vi "Lockin_sweep.vi"(0 "Transport":refnum<class "Transport.lvclass">, 3 "error in (no error)":errorcluster) -> (7 "Transport out":refnum<class "Transport.lvclass">, 10 "error out":errorcluster)   [LabVIEW 2019, in "Transport.lvclass"]
doc: "This VI uses the Lockin Sweep Method. That is, you tell the lockin to sweep from Start to End in a certain amount of time. The lockin will run independently while it executes the sweep. While the lockin is sweeping, this VI will poll the lockin once per second to get a snapshot of current results and the sweep status (sweeping or not sweeping). When the lockin is finished sweeping this VI will ask for the final sweep results and save them. The spacing between points is determined by the \"Fs Output\" control in the Lockin."
uses:
  Transport.lvclass
  Control Experiment/Control Experiment.lvclass
  <userlib>/LevyLab/Lockin-Multichannel/Instrument.DAQ/Typedefs/Sweep.Configuration--Cluster.ctl
  <userlib>/LevyLab/Lockin-Multichannel/Instrument.DAQ/Instrument.DAQ.lvclass
  <userlib>/LevyLab/Lockin-Multichannel/Instrument.DAQ/Typedefs/Sweep.Channel--Cluster.ctl
  <userlib>/LevyLab/Lockin-Multichannel/Instrument.Lockin/Instrument.Lockin.lvclass
  <userlib>/LevyLab/Lockin-Multichannel/Instrument.Lockin/Typedefs/Results Type--Enum.ctl
  <userlib>/LevyLab/Lockin-Multichannel/Instrument.DAQ/Typedefs/Sweep.Pattern--Enum.ctl
  <userlib>/LevyLab/Lockin-Multichannel/Instrument.DAQ/Typedefs/Sweep.Channel--Cluster--Array.ctl
  <vilib>/PRIrvin/XY Utilities/xy_utilities.lvlib
  217905a9-ad64-4e54-8703-31da4ffbd4c0.vi
  9896b5e5-a649-4b1b-acc0-fd49b17a1bc1.vi
  Typedefs/Lockin_Sweep JSON--Cluster.ctl
  <userlib>/LevyLab/Instrument Framework/Instrument Types/Cryostat/Typedefs/Magnet Axis--Enum.ctl
  <userlib>/LevyLab/Instrument Framework/Instrument Types/Cryostat/Instrument.Cryostat.lvclass
  <userlib>/LevyLab/Instrument Framework/Instrument Types/CBridge/Instrument.CBridge.lvclass
  <userlib>/LevyLab/Instrument Framework/Instrument Types/Strain/Instrument.Strain.lvclass
  C:/Program Files/National Instruments/LabVIEW 2019/user.lib/LevyLab/Instrument Framework/Instrument/Instrument.lvclass
  C:/Program Files/National Instruments/LabVIEW 2019/vi.lib/JKI/JKI SMO/SMO/SMO.lvclass
  <vilib>/PRIrvin/XY Utilities/subVIs/Divide float (multiple).vi
  <vilib>/PRIrvin/XY Utilities/subVIs/Multiply float (multiple).vi
  <vilib>/Utility/Data Type/NI_Data Type.lvlib
  <userlib>/LevyLab/Instrument Framework/Instrument/Instrument.lvclass
  <userlib>/LevyLab/Instrument Framework/Instrument Types/Lockin/Instrument.LockinAPI.lvclass
  <userlib>/LevyLab/Instrument Framework/Instrument Types/Amplifier/Instrument.Amplifier.lvclass
  <userlib>/LevyLab/Instrument Framework/Instrument Types/Delay Line/Instrument.DelayLine.lvclass
  <userlib>/LevyLab/Instrument Framework/Instrument Types/VNA/Instrument.VNA.lvclass
  <userlib>/LevyLab/Instrument Framework/Instrument Types/VSource/Instrument.VSource.lvclass
  Control Experiment/Typedefs/Instrument Types--enum.ctl
  Attributes/Instrument Attributes.lvlib
  ac72d6f7-f5c3-431a-8621-5120436d0f52.vi
  <userlib>/LevyLab/Debug/Debug.lvlib
  d7da78e6-7697-4005-8475-e4e7ed229128.vi
  C:/Program Files/National Instruments/LabVIEW 2019/user.lib/LevyLab/Instrument Framework/Instrument Types/Lockin/Instrument.LockinAPI.lvclass
panel:
  in  "stop":bool
  in  "Tab Control":T1(tab)
  in  "refresh (ms)":u32=1000
  out "state history":string
  out "Sweep Tables":cluster{"Ch":i32, "Table":dbl[]}[](array[cluster]) {"Table" format="%#_3p"; "Ch" min=1 max=16}
  in  "Emergency Stop Visible?":bool
  out "elapsed time (s)":i32=231
  out "Experiment Comments":string
  out "Experiment Folder":string
  out "time b/w points (ms)":u32=1037
  out "Sweep Channels":T2 {"Table" format="%#_1f"; "Channel" min=1 max=128; "Start" format="%#_6p"; "End" format="%#_6p"}
  out "Sweep Time (s)":dbl
  out "Initial Wait (s)":dbl
  out "Return to Start":bool
  out "Instrument Status":string
  in  "Emergency Stop 1":bool caption="Emergency Stop"
  out "Lockin (X)":cluster{"Wavenumber":dbl[], "Data":dbl[]}[](graph)
  out "Lockin (Y)":cluster{"Wavenumber":dbl[], "Data":dbl[]}[](graph)
  in  "Units":enum16{"ohms & siemens", "h/e2 & e2/h"}(ring)
  out "Resistance":cluster{"X-array":dbl[], "Y-array":dbl[]}[](graph)
  out "Conductance":cluster{"X-array":dbl[], "Y-array":dbl[]}[](graph)
  in  "Emergency Stop 2":bool caption="Emergency Stop"
  out "AI":cluster{"Wavenumber":dbl[], "Data":dbl[]}[](graph)
  out "AO":cluster{"Wavenumber":dbl[], "Data":dbl[]}[](graph)
  in  "Emergency Stop 3":bool caption="Emergency Stop"
  out "2 Terminal":cluster{"Wavenumber":dbl[], "Data":dbl[]}[](graph)
  out "4 Terminal":cluster{"Wavenumber":dbl[], "Data":dbl[]}[](graph)
  in  "Emergency Stop 4":bool caption="Emergency Stop"
  # "VI Configuration"
  # "Status"
  # "Experiment Configuration*"
  # "VI Description"
  # "Run a sweep on the lockin itself. The lockin is told to sweep from Start to End over a set time, and it runs the sweep on its own. While it sweeps, this VI polls the lockin once per fresh time for a snapshot of the current results and the sweep status. When the sweep finishes, it reads the final sweep results and saves them. The point spacing is set by the lockin's \"Fs Output\" control."
  # "*Change these values in Transport Server"
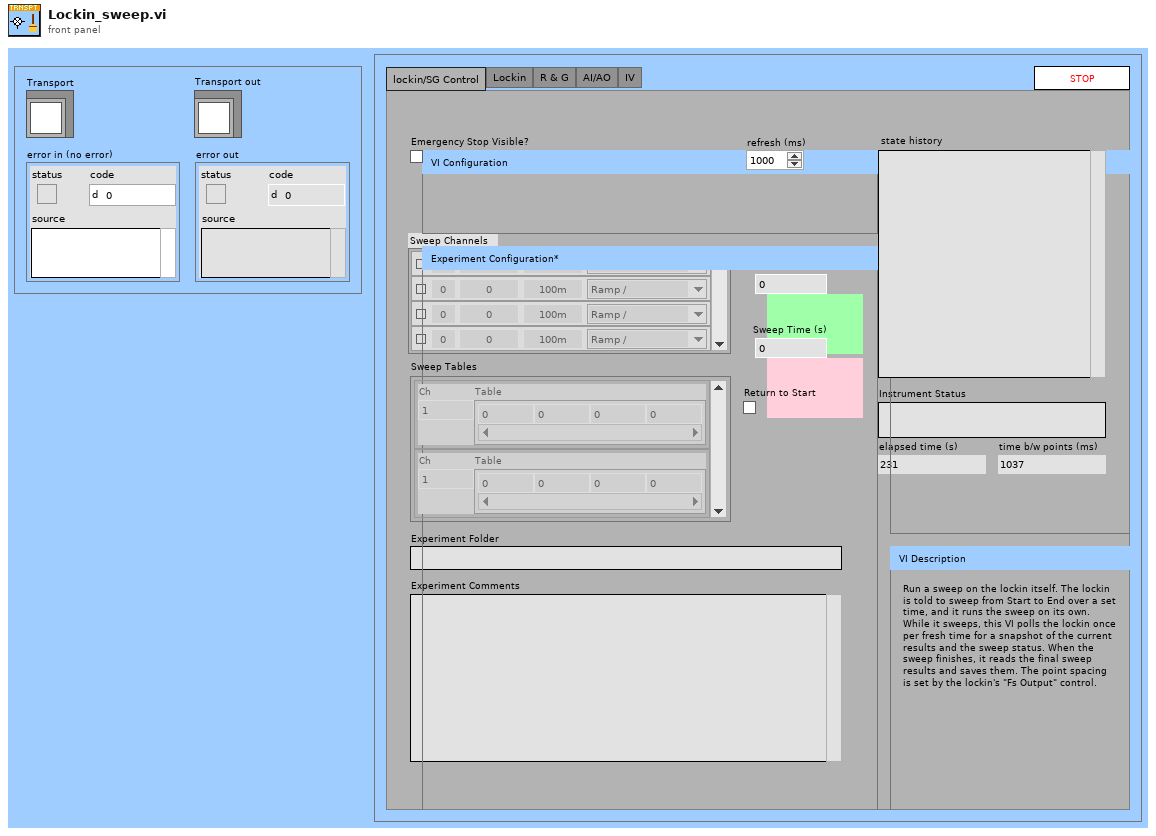
[diagram p1: front panel]
types:
  T1 = enum32{"lockin/SG Control", "Lockin", "R & G", "AI/AO", "IV"}
  T2 = typedef "Instrument.Lockin.lvlib/Instrument.DAQ.lvclass/Sweep.Channel--Cluster--Array.ctl" = T3[]
  T3 = typedef "Instrument.Lockin.lvlib/Instrument.DAQ.lvclass/Sweep.Channel--Cluster.ctl" = cluster{"Enable?":bool, "Channel":u16, "Start":dbl, "End":dbl, "Pattern":T4, "Table":dbl[]}
  T4 = typedef "Instrument.Lockin.lvlib/Instrument.DAQ.lvclass/Sweep.Pattern--Enum.ctl" = enum16{"Ramp /", "Ramp /\\", "Smooth Ramp _/", "Smooth Ramp _/\\_", "Table"}
  T5 = enum32{"Invalid", "Standard", "Closed", "Hidden", "Minimized", "Maximized"}
  T6 = enum32{"invalid app kind", "Development System", "Run Time System", "Student Edition", "Embedded LabVIEW", "Evaluation", "Custom"}
  T7 = enum32{"Bad", "Idle", "Run top level", "Running"}
  T8 = typedef "Control Experiment.lvclass/Instrument Types--enum.ctl" = enum16{"DAQ", "Amplifier", "Temperature", "Magnet", "Rotator", "Level", "Capacitance", "Delay Line", "Strain Cell", "VNA", "Source"}
  T9 = typedef "Instrument.Lockin.lvlib/Instrument.Lockin.lvclass/Results Type--Enum.ctl" = enum16{"X", "Y", "R", "Theta", "Mean"}
  T10 = typedef "Instrument.Lockin.lvlib/Instrument.DAQ.lvclass/Sweep.Configuration--Cluster.ctl" = cluster{"sweepTime":dbl, "initialWaitTime":dbl, "returnToStart":bool, "sweepChannels":T2}
  T11 = typedef "Instrument.Cryostat.lvclass/Magnet Axis--Enum.ctl" = enum16{"X", "Y", "Z"}
  T12 = typedef "Transport.lvclass/Lockin_Sweep JSON--Cluster.ctl" = cluster{"initialWaitTime":dbl, "sweepTime":dbl, "Return to Start":bool, "sweepChannels":cluster{"Enable?":bool, "Channel":u16, "Start":dbl, "End":dbl, "Pattern":enum16{"Ramp /", "Ramp /\\", "Smooth Ramp _/", "Smooth Ramp _/\\_", "Table"}, "Table":dbl[]}[], "sweepTables":cluster{"Ch":i32, "Table":dbl[]}[]}
  T13 = typedef "Control Experiment.lvclass/Instrument Classes--cluster.ctl" = cluster{"DAQ":refnum<class "Instrument.LockinAPI.lvclass">, "Amplifier":refnum<class "Instrument.Amplifier.lvclass">, "Temperature":refnum<class "Instrument.Cryostat.lvclass">, "Magnet":refnum<class "Instrument.Cryostat.lvclass">, "Rotator":refnum<class "Instrument.Cryostat.lvclass">, "Level":refnum<class "Instrument.Cryostat.lvclass">, "Capacitance":refnum<class "Instrument.CBridge.lvclass">, "Delay Line":refnum<class "Instrument.DelayLine.lvclass">, "Strain Cell":refnum<class "Instrument.Strain.lvclass">, "VNA":refnum<class "Instrument.VNA.lvclass">, "Source":refnum<class "Instrument.VSource.lvclass">}
  T14 = cluster{"Core":cluster{"Current VI Reference":refnum<vi>, "Close Panel on Exit?":bool}, "Transport":refnum<class "Transport.lvclass">, "C.E.":refnum<class "Control Experiment.lvclass">, "Instruments":T13, "Time":dbl, "Temperature":dbl, "Magnet":dbl, "Results (Dictionary)":cluster{"key":string, "value":dbl}[], "Sweep Value":dbl, "ms [0]":u32, "ms [i]":u32, "Execution:State":enum32{"Bad", "Idle", "Run top level", "Running"}, "AO Waveforrm":waveform(dbl)[], "AI Waveform":waveform(dbl)[], "Sweep_AO":waveform(dbl)[], "Sweep_AI":waveform(dbl)[], "Sweep_X":waveform(dbl)[], "Sweep_Y":waveform(dbl)[], "Amplitude":dbl[], "UI stop":bool}
  T15 = cluster{"Current VI Reference":refnum<vi>, "Close Panel on Exit?":bool}
  T16 = cluster{"I-":i32, "I+":i32, "V1-":i32, "V1+":i32, "I2-":i32, "I2+":i32, "V2-":i32, "V2+":i32}
  T17 = cluster{"Enable?":bool, "Channel":u16, "Start":dbl, "End":dbl, "Pattern":enum16{"Ramp /", "Ramp /\\", "Smooth Ramp _/", "Smooth Ramp _/\\_", "Table"}, "Table":dbl[]}[]
  T18 = typedef "Instrument.LockinAPI.lvclass/LockinAPI.getState.states--enum.ctl" = enum16{"idle", "created", "started", "stopped", "sweeping"}
  T19 = typedef "Instrument.Lockin.lvlib/Instrument.DAQ.lvclass/AO.Channel--Cluster--Array.ctl" = T20[]
  T20 = typedef "Instrument.Lockin.lvlib/Instrument.DAQ.lvclass/AO.Channel--Cluster.ctl" = cluster{"Enable?":bool, "Channel":i32, "Amplitude":dbl, "Offset":dbl, "Frequency":dbl, "Phase":dbl, "Function":T21, "Sweeping?":bool, "Limit AC":bool, "Limit DC?":bool, "Duty Cycle":bool}
  T21 = typedef "Instrument.Lockin.lvlib/Instrument.DAQ.lvclass/AO.Channel.Function--Enum.ctl" = enum16{"sine", "square", "triangle", "saw"}
  T22 = typedef "Instrument.LockinAPI.lvclass/LockinAPI.SweepData--Cluster.ctl" = cluster{"AO":waveform(dbl)[], "AI":waveform(dbl)[], "X":waveform(dbl)[], "Y":waveform(dbl)[]}
  T23 = typedef "LV-Data.lvclass/Dictionary--cluster.ctl" = cluster{"key":string, "value":variant}
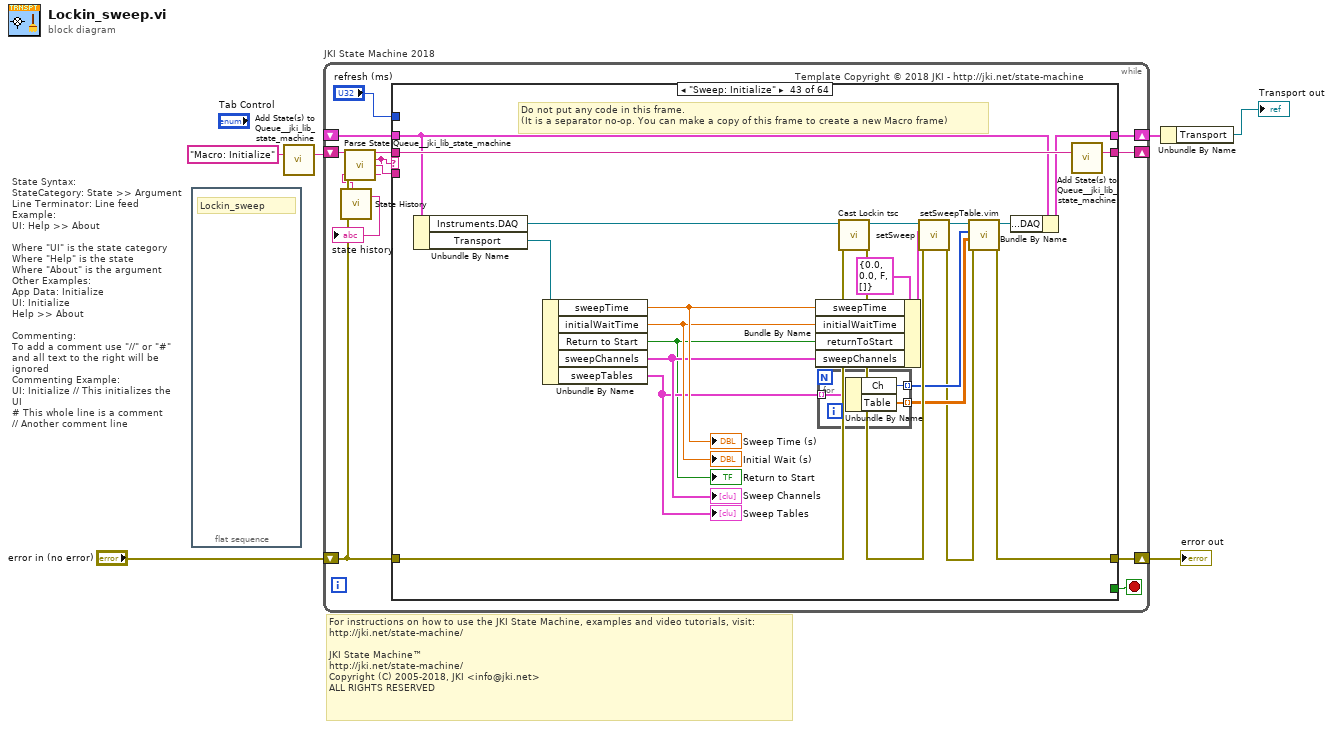
[diagram p0: block diagram]
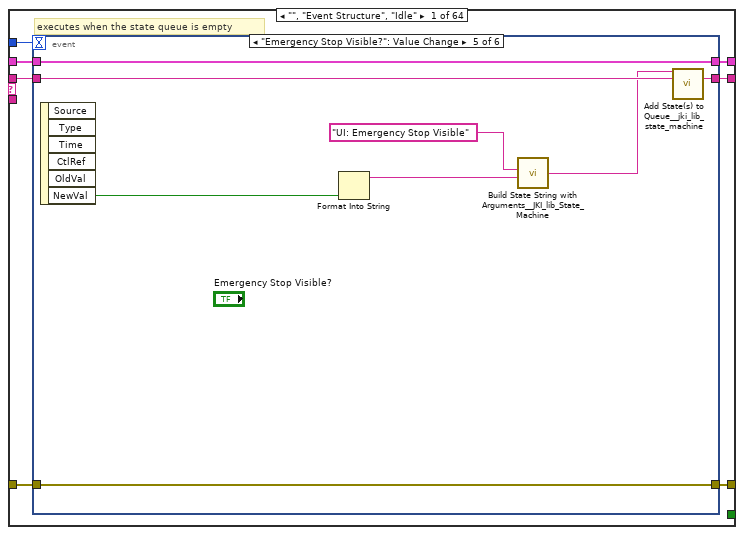
[diagram p2: hidden frame]
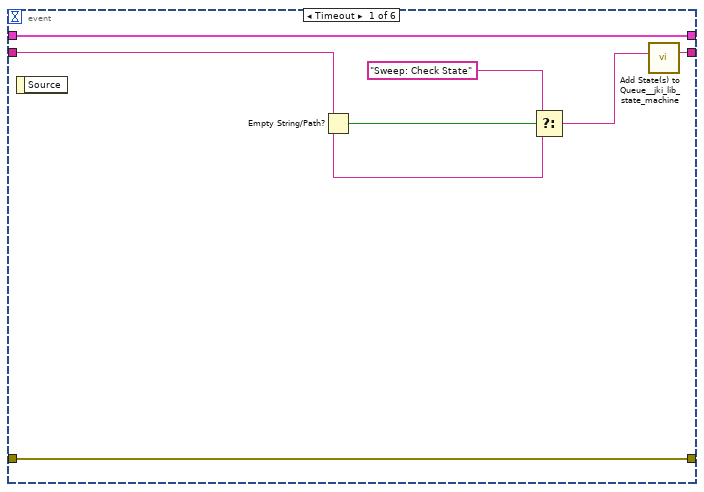
[diagram p3: hidden frame]
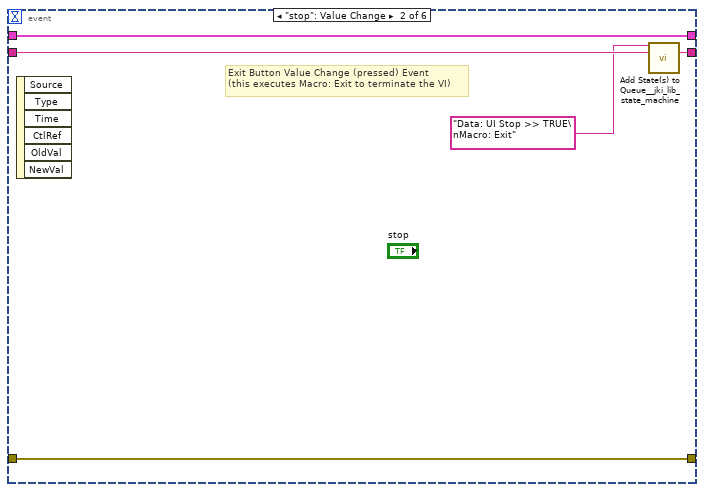
[diagram p4: hidden frame]
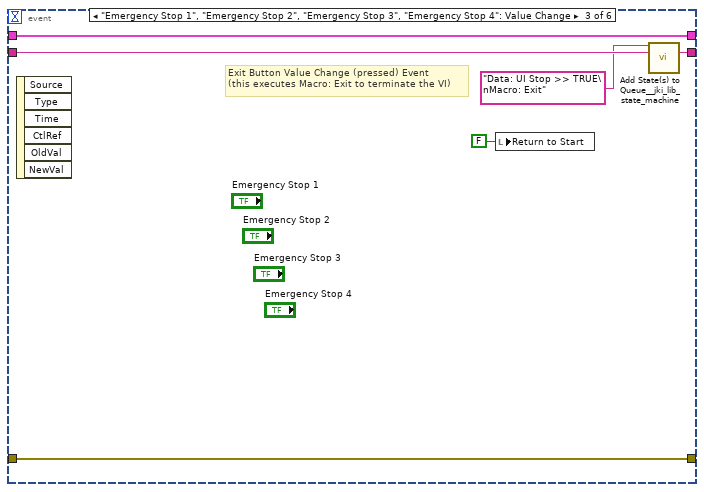
[diagram p5: hidden frame]
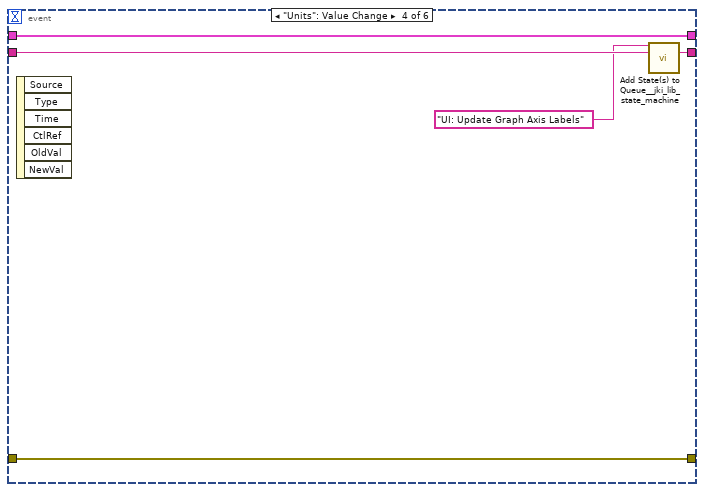
[diagram p6: hidden frame]
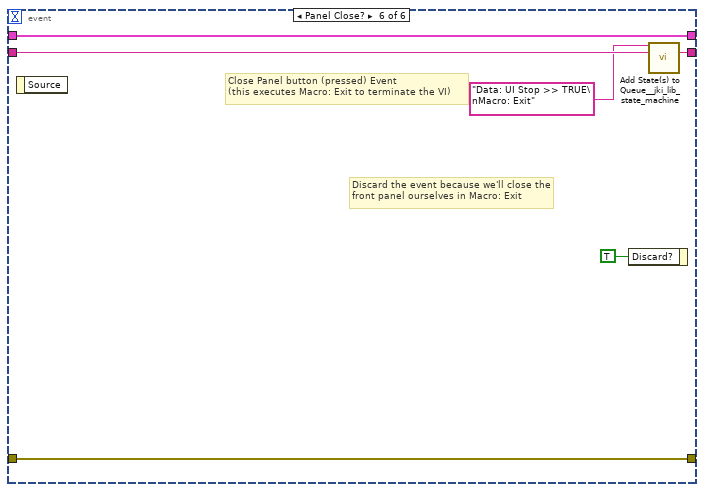
[diagram p7: hidden frame]
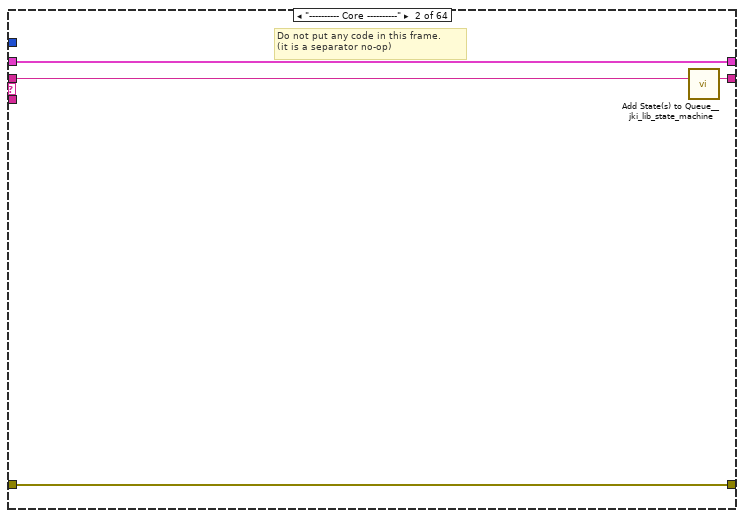
[diagram p8: hidden frame]
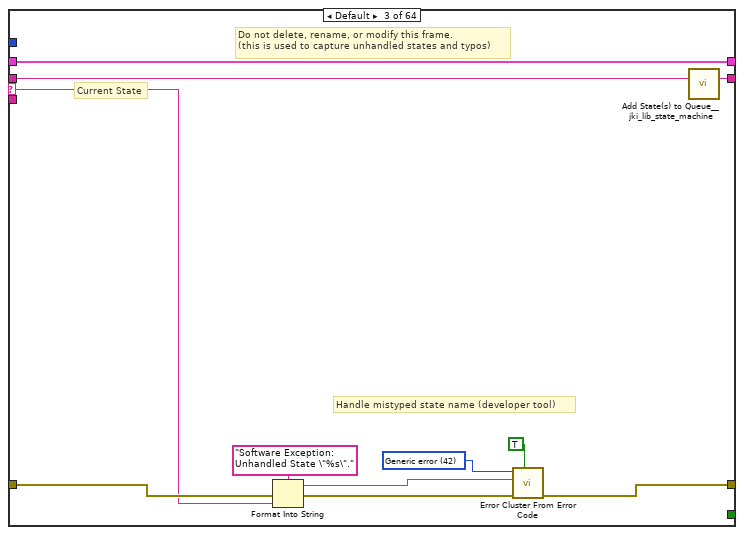
[diagram p9: hidden frame]
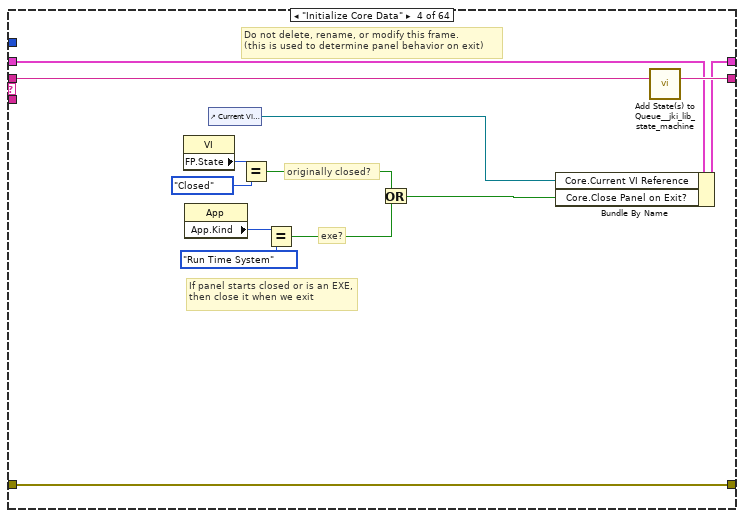
[diagram p10: hidden frame]
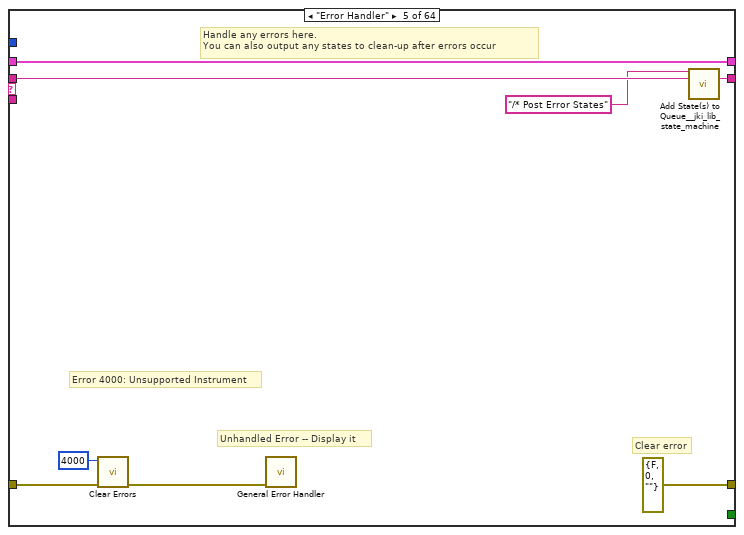
[diagram p11: hidden frame]
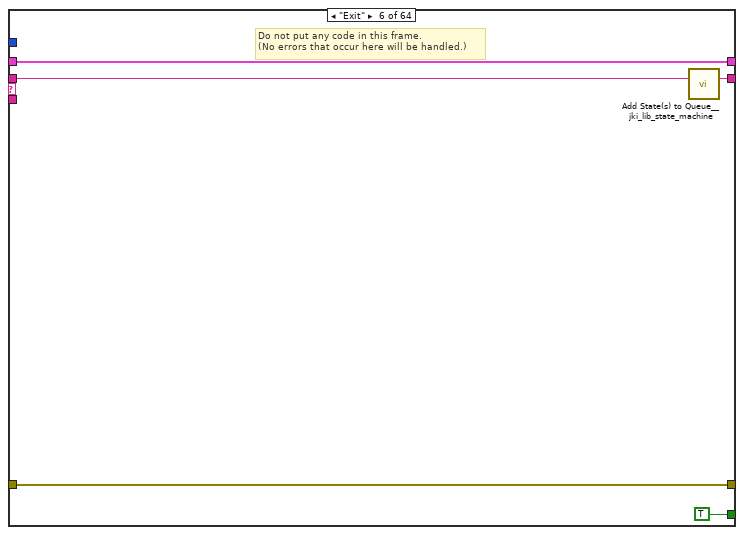
[diagram p12: hidden frame]
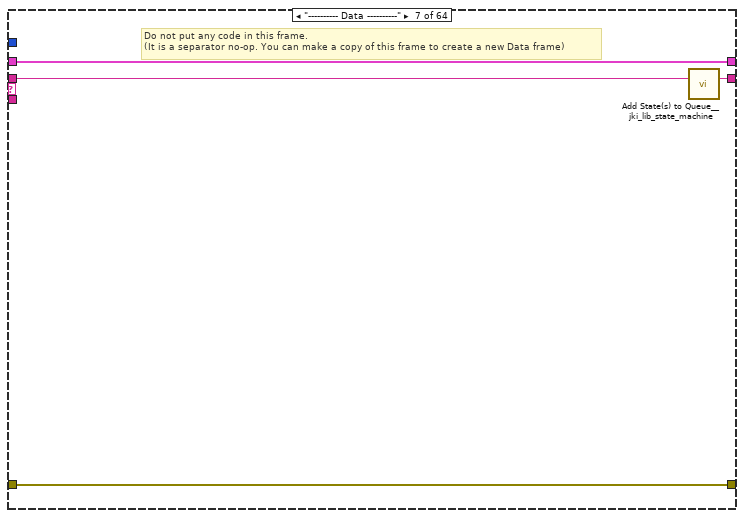
[diagram p13: hidden frame]
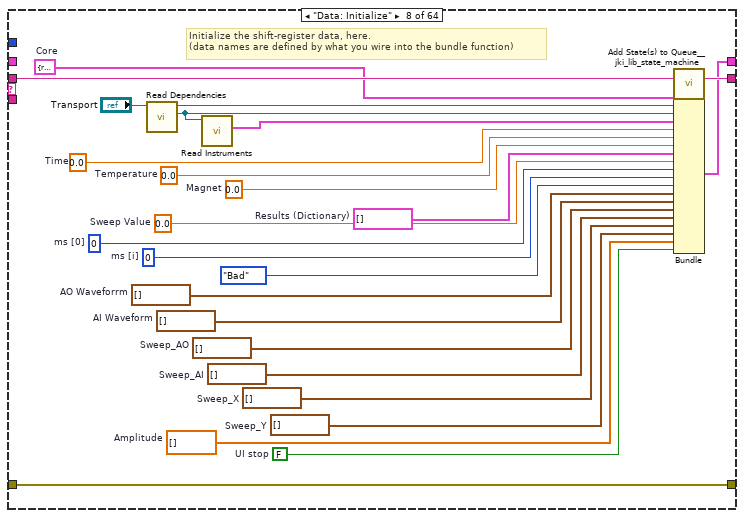
[diagram p14: hidden frame]
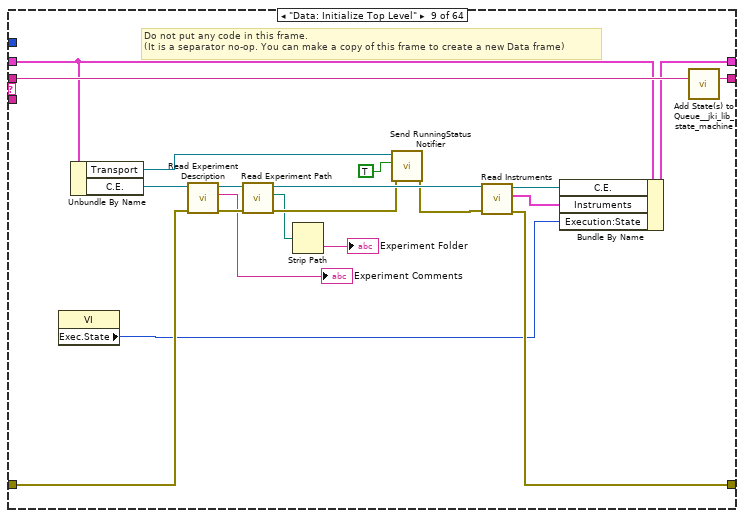
[diagram p15: hidden frame]
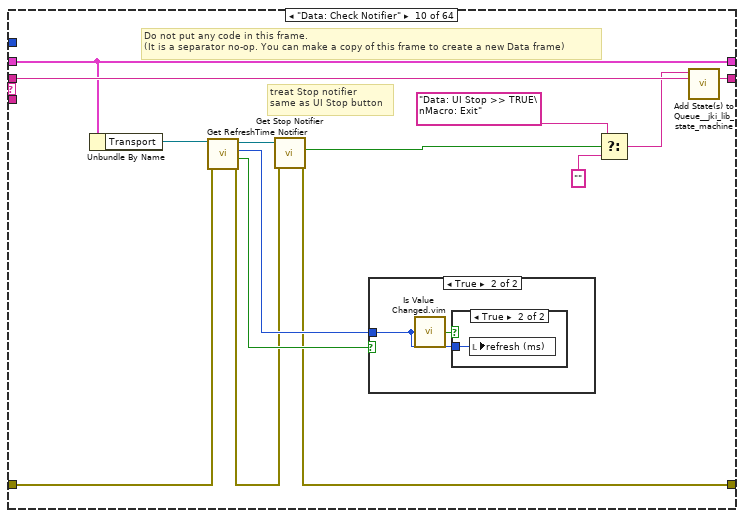
[diagram p16: hidden frame]
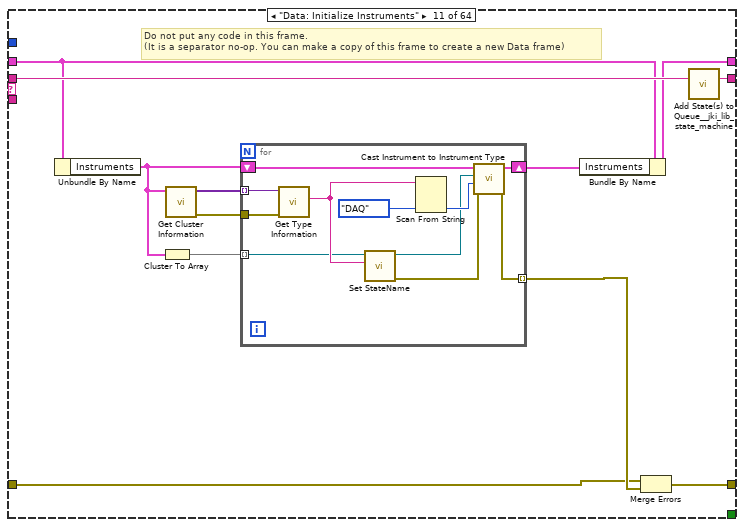
[diagram p19: hidden frame]
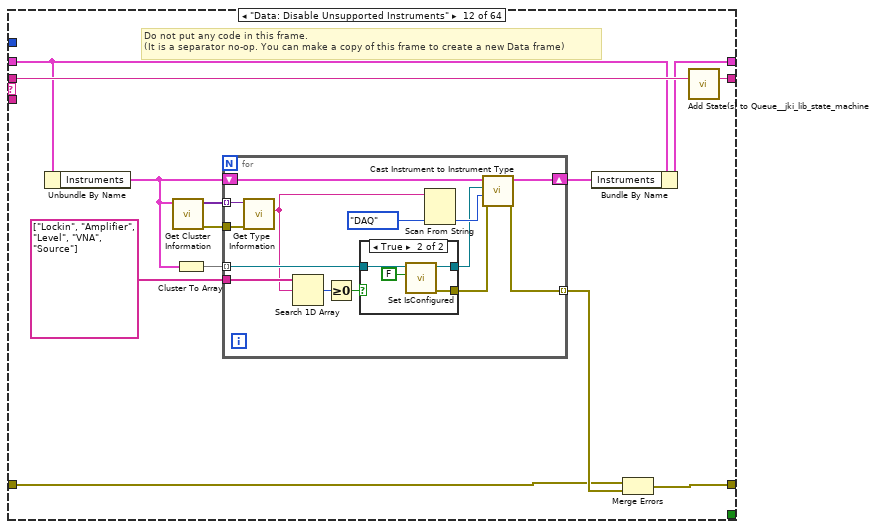
[diagram p20: hidden frame]
diagram:
  # "For instructions on how to use the JKI State Machine, examples and video tutorials, visit:\nhttp://jki.net/state-machine/\n\nJKI State Machine™\nhttp://jki.net/state-machine/\nCopyright (C) 2005-2018, JKI <info@jki.net>\nALL RIGHTS RESERVED"
  # "State Syntax:\nStateCategory: State >> Argument\nLine Terminator: Line feed\nExample:\nUI: Help >> About\n\nWhere \"UI\" is the state category\nWhere \"Help\" is the state\nWhere \"About\" is the argument\nOther Examples:\nApp Data: Initialize\nUI: Initialize\nHelp >> About\n\nCommenting:\nTo add a comment use \"//\" or \"#\" and all text to the right will be ignored\nCommenting Example:\nUI: Initialize // This initializes the UI\n# This whole line is a comment\n// Another comment line"
  n1 = flat-sequence {
    frame #0 {
      # "Lockin_sweep"
    }
  }
  n2 = call <vilib>:"Add State(s) to Queue__jki_lib_state_machine.vi"("State(s) in (\"\")"="Macro: Initialize") -> ("States Out"=w6:string)  [unwired: 14 in]
  n3 = while "JKI State Machine 2018" {
    shift-right: [w13] -> w4
    shift-left: _ -> [w12]
    shift-right: [w16] -> w2
    shift-left: "error in (no error)" -> [w11]
    shift-right: [w15] -> _
    shift-left: w6 -> [w10]
    stop <- w14 stop-if-true
    # "Template Copyright © 2018 JKI - http://jki.net/state-machine"
    n4 = call <vilib>:"Parse State Queue__jki_lib_state_machine.vi"("State Queue"=w10, "Error In (no error)"=w11) -> ("Remaining States"=w18:string, "Current State"=w9:string, "Arguments"=w17:string)  [unwired: 11 in]
    n5 = call <userlib>:"State History.vi"("Current State"=w9) -> ("History"=→"state history":string)  [unwired: 9 in, 1 out]
    n6 = case shown="\"Sweep: Initialize\"" w9 {
      selector: w9 -> [_ _ w67 _ _ _ _ _ _ _ _ _ _ _ _ _ _ _ _ _ _ _ _ _ _ _ _ _ _ _ _ _ _ _ _ _ _ _ _ _ _ _ _ _ _ _ _ _ _ _ _ _ _ _ _ _ _ _ _ _ _ _ _ _]
      tunnel: w18 -> [w25 w66 w71 w90 w98 w103 w107 w132 w152 w166 w181 w205 w236 w271 w283 w310 w331 w343 w353 w359 w370 w386 w401 w427 w444 w464 w502 w551 w576 w591 w609 w656 w668 w737 w742 w747 w760 w773 w778 w790 w801 w805 w827 w842 w854 w868 w892 w905 w909 w913 w924 w939 w961 w989 w1022 w1044 w1066 w1088 w1120 w1141 w1145 w1149 w1169 w1188]
      tunnel: w17 -> [_ _ _ _ _ _ _ _ _ _ _ _ _ _ _ w305 _ _ _ w354 w366 _ w388 _ _ _ _ w545 w565 _ _ _ w662 _ _ _ _ _ _ _ _ _ _ _ _ _ _ _ _ _ _ _ _ _ _ _ _ _ _ _ _ _ _ _]
      tunnel: w12 -> [w23 w63 w69 w83 w95 w101 w104 _ w142 w157 w178 w202 w233 w256 w277 w306 w325 w340 w344 w357 w367 w382 w398 w417 w440 w461 w499 w549 w568 w583 w606 w646 w664 w734 w738 w744 w756 w769 w774 w782 w798 w802 w824 w840 w848 w866 w890 w902 w907 w910 w917 w933 w954 w980 w1016 w1038 w1060 w1082 w1112 w1139 w1142 w1146 w1157 w1183]
      tunnel: [w22 w64 w73 w87 errorcluster {"status"=FALSE, "code"=0, "source"=""} ("error out") w100 w105 w129 w144 w155 w177 w195 w232 w258 w275 w308 w326 w341 w346 w355 w368 w378 w399 w422 w442 w462 w500 w548 w569 w589 w607 w637 w665 w735 w740 w745 w749 w771 w776 w788 w799 w803 w812 w835 w852 w861 w879 w903 w906 w911 w915 w927 w949 w978 w1009 w1032 w1054 w1076 w1118 w1136 w1143 w1147 w1160 w1181] -> w16
      tunnel: w11 -> [w21 w64 w72 w87 w92 w100 w105 w129 w145 w154 w170 w196 w231 w265 w278 w308 w317 w341 w351 w356 w368 w373 w399 w421 w438 w453 w486 w548 w563 w589 w607 w638 w666 w735 w740 w745 w748 w771 w776 w788 w799 w803 w818 w831 w843 w857 w869 w903 w906 w911 w916 w937 w956 w976 w1017 w1039 w1061 w1083 w1096 w1127 w1143 w1147 w1152 w1176]
      tunnel: [w24 w65 w70 w89 w97 w102 w106 w131 w151 w165 w180 w204 w235 w270 w282 w309 w330 w342 w352 w358 w369 w385 w400 w426 w443 w463 w501 w550 w575 w590 w608 w655 w667 w736 w741 w746 w759 w772 w777 w789 w800 w804 w826 w841 w853 w867 w891 w904 w908 w912 w923 w938 w960 w988 w1021 w1043 w1065 w1087 w1119 w1140 w1144 w1148 w1168 w1187] -> w15
      tunnel: [_ _ _ _ _ TRUE _ _ _ _ _ _ _ _ _ _ _ _ _ _ _ _ _ _ _ _ _ _ _ _ _ _ _ _ _ _ _ _ _ _ _ _ _ _ _ _ _ _ _ _ _ _ _ _ _ _ _ _ _ _ _ _ _ _] -> w14
      tunnel: [w20 w63 w69 w88 w95 w101 w104 w130 w143 w157 w179 w203 w234 w266 w276 w307 w328 w340 w347 w357 w367 w381 w398 w417 w440 w461 w499 w549 w568 w583 w606 w646 w664 w734 w738 w744 w756 w769 w774 w782 w798 w802 w825 w839 w849 w865 w889 w902 w907 w910 w921 w936 w959 w981 w1020 w1042 w1064 w1086 w1111 w1138 w1142 w1146 w1158 w1184] -> w13
      tunnel: "refresh (ms)" -> [w19 _ _ _ _ _ _ _ _ _ _ _ _ _ _ _ _ _ _ _ _ _ _ _ _ _ _ _ _ _ _ _ _ _ _ _ _ _ _ _ _ _ _ _ _ _ _ _ _ _ _ _ _ _ _ _ _ _ _ _ _ _ _ _]
      frame "", "Event Structure", "Idle" {
        # "executes when the state queue is empty"
        n7 = event shown="[4] \"Emergency Stop Visible?\": Value Change" {
          selector: _ -> [_ _ _ _ _ _]
          dyn-events: _ -> [_ _ _ _ _ _]
          timeout: w19 -> [_ _ _ _ _ _]
          tunnel: w25 -> [w27 w37 w43 w48 w56 w62]
          tunnel: [w32 w36 w42 w47 w55 w61] -> w24
          tunnel: w23 -> [w30 w33 w40 w45 w53 w59]
          tunnel: [w31 w35 w41 w46 w54 w60] -> w22
          tunnel: w21 -> [w31 w35 w41 w46 w54 w60]
          tunnel: [w30 w33 w40 w45 w53 w59] -> w20
          event Timeout {
            n8 = event-data() -> ()  [unwired: 1 in, 1 out]
            n9 = Empty String/Path?(string/path=w27) -> (empty?=w29:bool)
            n10 = Select(t="Sweep: Check State" ("State(s) in Front (\"\")"), s=w29, f=w27) -> (s? t:f=w28:string)
            n11 = call <vilib>:"Add State(s) to Queue__jki_lib_state_machine.vi"("State(s) in (\"\")"=w28) -> ("States Out"=w32:string)  [unwired: 14 in]
          }
          event "stop": Value Change {
            # "Exit Button Value Change (pressed) Event\n(this executes Macro: Exit to terminate the VI)"
            n12 = event-data() -> ()  [unwired: 1 in, 6 out]
            n13 = call <vilib>:"Add State(s) to Queue__jki_lib_state_machine.vi"("State(s) in Front (\"\")"="Data: UI Stop >> TRUE\nMacro: Exit", "State(s) in (\"\")"=w37) -> ("States Out"=w36:string)  [unwired: 13 in]
          }
          event "Emergency Stop 1", "Emergency Stop 2", "Emergency Stop 3", "Emergency Stop 4": Value Change {
            # "Exit Button Value Change (pressed) Event\n(this executes Macro: Exit to terminate the VI)"
            n14 = event-data() -> ()  [unwired: 1 in, 6 out]
            n15 = local write "Return to Start"(FALSE ("Return to Start")) -> ()
            n16 = call <vilib>:"Add State(s) to Queue__jki_lib_state_machine.vi"("State(s) in Front (\"\")"="Data: UI Stop >> TRUE\nMacro: Exit", "State(s) in (\"\")"=w43) -> ("States Out"=w42:string)  [unwired: 13 in]
          }
          event "Units": Value Change {
            n17 = event-data() -> ()  [unwired: 1 in, 6 out]
            n18 = call <vilib>:"Add State(s) to Queue__jki_lib_state_machine.vi"("State(s) in Front (\"\")"="UI: Update Graph Axis Labels", "State(s) in (\"\")"=w48) -> ("States Out"=w47:string)  [unwired: 13 in]
          }
          event "Emergency Stop Visible?": Value Change {
            n19 = event-data() -> ("NewVal"=w50:bool)  [unwired: 1 in, 5 out]
            n20 = Format Into String(w50) -> (resulting string=w52:string)  [unwired: 3 in, 1 out]
            n21 = call <vilib>:"Build State String with Arguments__JKI_lib_State_Machine.vi"("Arguments (\"\")"=w52, "State"="UI: Emergency Stop Visible") -> ("State with Arguments"=w49:string)  [unwired: 4 in]
            n22 = call <vilib>:"Add State(s) to Queue__jki_lib_state_machine.vi"("State(s) in Front (\"\")"=w49, "State(s) in (\"\")"=w56) -> ("States Out"=w55:string)  [unwired: 13 in]
          }
          event Panel Close? {
            # "Discard the event because we'll close the front panel ourselves in Macro: Exit"
            # "Close Panel button (pressed) Event\n(this executes Macro: Exit to terminate the VI)"
            n23 = event-data() -> ()  [unwired: 1 in, 1 out]
            n24 = event-data("Discard?"=TRUE) -> ()  [unwired: 1 in, 1 out]
            n25 = call <vilib>:"Add State(s) to Queue__jki_lib_state_machine.vi"("State(s) in Front (\"\")"="Data: UI Stop >> TRUE\nMacro: Exit", "State(s) in (\"\")"=w62) -> ("States Out"=w61:string)  [unwired: 13 in]
          }
        }
      }
      frame "---------- Core ----------" {
        # "Do not put any code in this frame.\n(it is a separator no-op)"
        n26 = call <vilib>:"Add State(s) to Queue__jki_lib_state_machine.vi"("State(s) in (\"\")"=w66) -> ("States Out"=w65:string)  [unwired: 14 in]
      }
      frame Default {
        w76 = 42 items=["No error", "Argument error", "Memory is full", "Out of zone", "End of file", "File already open", "Generic file I/O error", "File not found", "File permission error", "Disk is full", "Duplicate path", "Too many files open", "System feature not enabled", "Resource file not found", "Cannot add resource", "Resource not found", "Image not found", "Image memory error", "Pen does not exist", "Config type invalid", "Config token not found", "Config parse error", "Config memory error", "Bad external code format", "Bad external code offset", "External code not present", "Null window", "Destroy window error", "Null menu", "Print aborted", "Bad print record", "Print driver error", "Windows error during printing", "Memory error during printing", "Print dialog error", "Generic print error", "Invalid device refnum", "Device not found", "Device parameter error", "Device unit error", "Cannot open device", "Device call aborted", "Generic error", "Cancelled by user", "Object ID too low", "Object ID too high", "Object not in heap", "Unknown heap", "Unknown object (invalid DefProc)", "Unknown object (DefProc not in table)", "Message out of range", "Invalid (null) method", "Unknown message", "Manager call not supported", "Bad address", "Network operation in progress", "Network operation timed out", "Connection is busy", "Network attribute not supported", "Network error", "Address in use", "System out of memory", "Connection aborted", "Connection refused", "Not connected", "Already connected", "Connection closed", "Initialization error (interapplication manager)", "Bad occurrence", "Wait on unbound occurrence handler", "Occurrence queue overflow", "Datalog type conflict", "Unused", "Unrecognized type (interapplication manager)", "Memory corrupt", "Failed to make temporary DLL", "Old CIN version", "Drag socket not found", "Failed to load drop-object", "Failed to register OLE object", "Failed to release OLE object", "Format specifier type mismatch", "Unknown format specifier", "Too few format specifiers", "Too many format specifiers", "Scan failed", "Newer CIN version", "Error converting to variant", "Runtime menu error", "Password tampered", "Variant attribute not found", "Incompatible variant data type", "Event data is not available", "Event Store is not present", "Occurrence is not found", "Event Queue is not created", "Event info is not available", "Refnum passed is NULL", "Error retrieving Class GUID", "Error retrieving CoClass GUID", "Error retrieving TypeLib GUID.", "Bad built application magic bytes.", "Specific driver is different from the specific driver associated with the Logical Name.", "There is no session opened to the class driver.", "Max Error", "MAX - Error with config objects", "MAX - Error loading configuration", "MAX - Group not supported"]
        # "Current State"
        # "Do not delete, rename, or modify this frame.\n(this is used to capture unhandled states and typos)"
        # "Handle mistyped state name (developer tool)"
        n27 = Format Into String(format string="Software Exception: Unhandled State \"%s\"." ("message"), error in=w72, w67) -> (resulting string=w75:string, error out=w74:errorcluster)  [unwired: 1 in]
        n28 = call <vilib>:"Error Cluster From Error Code.vi"("show call chain? (False)"=TRUE, "error in (no error)"=w74, "error message (\"\")"=w75, "error code (0)"=w76) -> ("error out"=w73:errorcluster)  [unwired: 5 in]
        n29 = call <vilib>:"Add State(s) to Queue__jki_lib_state_machine.vi"("State(s) in (\"\")"=w71) -> ("States Out"=w70:string)  [unwired: 14 in]
      }
      frame "Initialize Core Data" {
        # "Do not delete, rename, or modify this frame.\n(this is used to determine panel behavior on exit)"
        # "originally closed?"
        # "exe?"
        # "If panel starts closed or is an EXE, then close it when we exit"
        n30 = property class="VI"() -> ("FP.State"=w80:T5)  [unwired: 2 in, 2 out]
        n31 = property class="App"() -> ("App.Kind"=w86:T6)  [unwired: 2 in, 2 out]
        n32 = control-ref of="Current VI Reference"() -> (w81:refnum<vi>)
        n33 = Equal?(x=w80, y=T5."Closed" ("Front Panel Window:State")) -> (x = y?=w78:bool)
        n34 = Equal?(x=w86, y=T6."Run Time System" ("Application:Kind")) -> (x = y?=w84:bool)
        n35 = Or(x=w78, y=w84) -> (x .or. y?=w82:bool)
        n36 = Bundle By Name(cluster=w83, "Core.Current VI Reference"=w81, "Core.Close Panel on Exit?"=w82) -> (w88:T14)
        n37 = call <vilib>:"Add State(s) to Queue__jki_lib_state_machine.vi"("State(s) in (\"\")"=w90) -> ("States Out"=w89:string)  [unwired: 14 in]
      }
      frame "Error Handler" {
        # "Error 4000: Unsupported Instrument"
        # "Unhandled Error -- Display it"
        # "Handle any errors here.\nYou can also output any states to clean-up after errors occur"
        # "Clear error"
        n38 = call <vilib>:"Clear Errors.vi"("error in (no error)"=w92, "specific error code to clear (0: all)"=4000) -> ("error out"=w91:errorcluster)  [unwired: 4 in, 1 out]
        n39 = call <vilib>:"General Error Handler.vi"("error in (no error)"=w91) -> ()  [unwired: 10 in, 5 out]
        n40 = call <vilib>:"Add State(s) to Queue__jki_lib_state_machine.vi"("State(s) in Front (\"\")"="/* Post Error States", "State(s) in (\"\")"=w98) -> ("States Out"=w97:string)  [unwired: 13 in]
      }
      frame "Exit" {
        # "Do not put any code in this frame.\n(No errors that occur here will be handled.)"
        n41 = call <vilib>:"Add State(s) to Queue__jki_lib_state_machine.vi"("State(s) in (\"\")"=w103) -> ("States Out"=w102:string)  [unwired: 14 in]
      }
      frame "---------- Data ----------" {
        # "Do not put any code in this frame.\n(It is a separator no-op. You can make a copy of this frame to create a new Data frame)"
        n42 = call <vilib>:"Add State(s) to Queue__jki_lib_state_machine.vi"("State(s) in (\"\")"=w107) -> ("States Out"=w106:string)  [unwired: 14 in]
      }
      frame "Data: Initialize" {
        w109 = FALSE  # UI stop
        w112 = dbl[] []  # Amplitude
        w116 = waveform(dbl)[] []  # Sweep_Y
        w117 = waveform(dbl)[] []  # Sweep_X
        w113 = cluster{"key":string, "value":dbl}[] []  # Results (Dictionary)
        w119 = waveform(dbl)[] []  # Sweep_AO
        w118 = waveform(dbl)[] []  # Sweep_AI
        w120 = waveform(dbl)[] []  # AI Waveform
        w121 = waveform(dbl)[] []  # AO Waveforrm
        w122 = 0.0  # Sweep Value
        w123 = u32 0  # ms [i]
        w124 = u32 0  # ms [0]
        w126 = 0.0  # Time
        w127 = 0.0  # Magnet
        w125 = 0.0  # Temperature
        w128 = T15 {"Current VI Reference"=refnum, "Close Panel on Exit?"=FALSE}  # Core
        # "Initialize the shift-register data, here.\n(data names are defined by what you wire into the bundle function)"
        n43 = call "Read Dependencies.vi"("Transport"="Transport") -> ("C.E."=w111:refnum<class "Control Experiment.lvclass">, "Transport"=w114:refnum<class "Transport.lvclass">)  [unwired: 8 in, 1 out]
        n44 = call "Read Instruments.vi"("Control Experiment in"=w111) -> ("Instruments"=w110:T13)  [unwired: 8 in, 2 out]
        n45 = call <vilib>:"Add State(s) to Queue__jki_lib_state_machine.vi"("State(s) in (\"\")"=w132) -> ("States Out"=w131:string)  [unwired: 14 in]
        n46 = Bundle("Core"=w128, "Transport"=w114, "C.E."=w111, "Instruments"=w110, "Time"=w126, "Temperature"=w125, "Magnet"=w127, "Results (Dictionary)"=w113, "Sweep Value"=w122, "ms [0]"=w124, "ms [i]"=w123, "Execution:State"=T7."Bad", "AO Waveforrm"=w121, "AI Waveform"=w120, "Sweep_AO"=w119, "Sweep_AI"=w118, "Sweep_X"=w117, "Sweep_Y"=w116, "Amplitude"=w112, "UI stop"=w109) -> (w130:T14)  [unwired: 1 in]
      }
      frame "Data: Initialize Top Level" {
        # "Do not put any code in this frame.\n(It is a separator no-op. You can make a copy of this frame to create a new Data frame)"
        n47 = property class="VI"() -> ("Exec.State"=w141:T7)  [unwired: 2 in, 2 out]
        n48 = Unbundle By Name(w142) -> ("Transport"=w140:refnum<class "Transport.lvclass">, "C.E."=w146:refnum<class "Control Experiment.lvclass">)
        n49 = call "Read Experiment Description.vi"("error in (no error)"=w145, "Control Experiment in"=w146) -> ("error out"=w139:errorcluster, "Experiment Description"=→"Experiment Comments":string, "Control Experiment out"=w138:refnum<class "Control Experiment.lvclass">)  [unwired: 7 in]
        n50 = call "Read Experiment Path.vi"("error in (no error)"=w139, "Control Experiment in"=w138) -> ("error out"=w136:errorcluster, "Experiment Path"=w133:path, "Control Experiment out"=w148:refnum<class "Control Experiment.lvclass">)  [unwired: 7 in]
        n51 = Strip Path(path=w133) -> (name=→"Experiment Folder":string)  [unwired: 1 out]
        n52 = call "Send RunningStatus Notifier.vi"("error in (no error)"=w136, "Running?"=TRUE, "Transport in"=w140) -> ("error out"=w147:errorcluster)  [unwired: 7 in, 1 out]
        n53 = call "Read Instruments.vi"("error in (no error)"=w147, "Control Experiment in"=w148) -> ("error out"=w144:errorcluster, "Instruments"=w150:T13, "Control Experiment out"=w149:refnum<class "Control Experiment.lvclass">)  [unwired: 7 in]
        n54 = Bundle By Name(cluster=w142, "C.E."=w149, "Instruments"=w150, "Execution:State"=w141) -> (w143:T14)
        n55 = call <vilib>:"Add State(s) to Queue__jki_lib_state_machine.vi"("State(s) in (\"\")"=w152) -> ("States Out"=w151:string)  [unwired: 14 in]
      }
      frame "Data: Check Notifier" {
        # "treat Stop notifier\nsame as UI Stop button"
        # "Do not put any code in this frame.\n(It is a separator no-op. You can make a copy of this frame to create a new Data frame)"
        n56 = Unbundle By Name(w157) -> ("Transport"=w161:refnum<class "Transport.lvclass">)
        n57 = call "Get RefreshTime Notifier.vi"("error in (no error)"=w154, "Transport in"=w161) -> ("error out"=w156:errorcluster, "valid?"=w158:bool, "RefreshTime (ms)"=w159:u32, "Transport out"=w160:refnum<class "Transport.lvclass">)  [unwired: 6 in]
        n58 = call "Get Stop Notifier.vi"("error in (no error)"=w156, "Transport in"=w160) -> ("error out"=w155:errorcluster, "Stop?"=w153:bool)  [unwired: 7 in, 1 out]
        n59 = case shown="True" w158 {
          tunnel: w159 -> [_ w167]
          frame False {
          }
          frame True {
            n60 = call "Is Value Changed.vim"("value"=w167) -> ("changed or first call?"=w168:bool)
            n61 = case shown="True" w168 {
              tunnel: w167 -> [_ w169]
              frame False {
              }
              frame True {
                n62 = local write "refresh (ms)"(w169) -> ()
              }
            }
          }
        }
        n63 = Select(t="Data: UI Stop >> TRUE\nMacro: Exit", s=w153, f="") -> (s? t:f=w162:string)
        n64 = call <vilib>:"Add State(s) to Queue__jki_lib_state_machine.vi"("State(s) in Front (\"\")"=w162, "State(s) in (\"\")"=w166) -> ("States Out"=w165:string)  [unwired: 13 in]
      }
      frame "Data: Initialize Instruments" {
        # "Do not put any code in this frame.\n(It is a separator no-op. You can make a copy of this frame to create a new Data frame)"
        n65 = Unbundle By Name(w178) -> ("Instruments"=w171:T13)
        n66 = Cluster To Array(cluster=w171) -> (array=w176:refnum<class "Instrument.lvclass">[])
        n67 = call <vilib>:"Get Cluster Information.vi"("variant"=w171) -> ("error out"=w174:errorcluster, "cluster elements"=w175:variant[])  [unwired: 9 in]
        n68 = for {
          tunnel: w176 -> [w182] mode=indexing
          tunnel: [w190] -> w173 mode=indexing
          shift-right: [w191] -> w172
          shift-left: w171 -> [w192]
          tunnel: w175 -> [w187] mode=indexing
          tunnel: w174 -> [w186]
          n69 = call <vilib>:"Get Type Information.vi"("error in (no error)"=w186, "variant"=w187) -> ("name"=w183:string)  [unwired: 5 in, 4 out]
          n70 = call "Set StateName.vi"("StateName"=w183, "SMO"=w182) -> ("error out"=w184:errorcluster, "SMO out"=w185:refnum<class "Instrument.lvclass">)  [unwired: 8 in]
          n71 = Scan From String(input string=w183, default 1=Instrument_Types--enum."DAQ" ("Type")) -> (output 1=w188:T8)  [unwired: 3 in, 3 out]
          n72 = call "Cast Instrument to Instrument Type.vi"("error in (no error)"=w184, "Type"=w188, "Instrument in"=w185, "Instrument Classes"=w192) -> ("error out"=w190:errorcluster, "Instrument Classes out"=w191:T13)  [unwired: 5 in, 1 out]
        }
        n73 = Bundle By Name(cluster=w178, "Instruments"=w172) -> (w179:T14)
        n74 = Merge Errors(w170, w173) -> (w177:errorcluster)
        n75 = call <vilib>:"Add State(s) to Queue__jki_lib_state_machine.vi"("State(s) in (\"\")"=w181) -> ("States Out"=w180:string)  [unwired: 14 in]
      }
      frame "Data: Disable Unsupported Instruments" {
        # "Do not put any code in this frame.\n(It is a separator no-op. You can make a copy of this frame to create a new Data frame)"
        n76 = Unbundle By Name(w202) -> ("Instruments"=w194:T13)
        n77 = call <vilib>:"Get Cluster Information.vi"("variant"=w194) -> ("error out"=w199:errorcluster, "cluster elements"=w200:variant[])  [unwired: 9 in]
        n78 = Cluster To Array(cluster=w194) -> (array=w201:refnum<class "Instrument.lvclass">[])
        n79 = for {
          tunnel: w201 -> [w212] mode=indexing
          tunnel: [w217] -> w198 mode=indexing
          shift-right: [w218] -> w193
          shift-left: w194 -> [w219]
          tunnel: w200 -> [w214] mode=indexing
          tunnel: w199 -> [w213]
          tunnel: string[] ["Lockin", "Amplifier", "Level", "VNA", "Source"] ("element") -> [w209]
          n80 = call <vilib>:"Get Type Information.vi"("error in (no error)"=w213, "variant"=w214) -> ("name"=w208:string)  [unwired: 5 in, 4 out]
          n81 = Search 1D Array(1D array=w209, element=w208) -> (index of element=w206:i32)  [unwired: 1 in]
          n82 = Greater Or Equal To 0?(x=w206) -> (x >= 0?=w207:bool)
          n83 = case shown="True" w207 {
            tunnel: w212 -> [w220 w224]
            tunnel: [w220 w223] -> w211
            tunnel: [_ w222] -> w210
            frame False {
            }
            frame True {
              n84 = call "Set IsConfigured.vi"("IsConfigured?"=FALSE, "SMO"=w224) -> ("error out"=w222:errorcluster, "SMO out"=w223:refnum<class "Instrument.lvclass">)  [unwired: 8 in]
            }
          }
          n85 = Scan From String(input string=w208, default 1=Instrument_Types--enum."DAQ" ("Type")) -> (output 1=w215:T8)  [unwired: 3 in, 3 out]
          n86 = call "Cast Instrument to Instrument Type.vi"("error in (no error)"=w210, "Type"=w215, "Instrument in"=w211, "Instrument Classes"=w219) -> ("error out"=w217:errorcluster, "Instrument Classes out"=w218:T13)  [unwired: 5 in, 1 out]
        }
        n87 = Bundle By Name(cluster=w202, "Instruments"=w193) -> (w203:T14)
        n88 = Merge Errors(w196, w198) -> (w195:errorcluster)
        n89 = call <vilib>:"Add State(s) to Queue__jki_lib_state_machine.vi"("State(s) in (\"\")"=w205) -> ("States Out"=w204:string)  [unwired: 14 in]
      }
      frame "Data: Open Instruments" {
        # "Do not put any code in this frame.\n(It is a separator no-op. You can make a copy of this frame to create a new Data frame)"
        n90 = Unbundle By Name(w233) -> ("Instruments"=w227:T13)
        n91 = call <vilib>:"Get Cluster Information.vi"("variant"=w227) -> ("error out"=w228:errorcluster, "cluster elements"=w229:variant[])  [unwired: 9 in]
        n92 = Cluster To Array(cluster=w227) -> (array=w230:refnum<class "Instrument.lvclass">[])
        n93 = for {
          tunnel: w230 -> [w240] mode=indexing
          tunnel: [w246] -> w225 mode=indexing
          shift-right: [w249] -> w226
          shift-left: w227 -> [w250]
          tunnel: w229 -> [w243] mode=indexing
          tunnel: w228 -> [w241]
          n94 = call <vilib>:"Get Type Information.vi"("error in (no error)"=w241, "variant"=w243) -> ("name"=w242:string)  [unwired: 5 in, 4 out]
          n95 = call "Get IsConfigured.vi"("SMO"=w240) -> ("error out"=w237:errorcluster, "IsConfigured?"=w238:bool, "SMO out"=w239:refnum<class "Instrument.lvclass">)  [unwired: 8 in]
          n96 = case shown="True" w238 {
            tunnel: [_ w255] -> w247
            tunnel: w239 -> [w251 w254]
            tunnel: [w251 w253] -> w248
            tunnel: w237 -> [_ w252]
            frame False {
            }
            frame True {
              n97 = call-dynamic "Open.vi"("error in (no error)"=w252, "Instrument in"=w254) -> ("error out"=w255:errorcluster, "Instrument out"=w253:refnum<class "Instrument.lvclass">)  [unwired: 8 in]
            }
          }
          n98 = Scan From String(input string=w242, default 1=Instrument_Types--enum."DAQ" ("Type")) -> (output 1=w244:T8)  [unwired: 3 in, 3 out]
          n99 = call "Cast Instrument to Instrument Type.vi"("error in (no error)"=w247, "Type"=w244, "Instrument in"=w248, "Instrument Classes"=w250) -> ("error out"=w246:errorcluster, "Instrument Classes out"=w249:T13)  [unwired: 5 in, 1 out]
        }
        n100 = Bundle By Name(cluster=w233, "Instruments"=w226) -> (w234:T14)
        n101 = Merge Errors(w231, w225) -> (w232:errorcluster)
        n102 = call <vilib>:"Add State(s) to Queue__jki_lib_state_machine.vi"("State(s) in (\"\")"=w236) -> ("States Out"=w235:string)  [unwired: 14 in]
      }
      frame "Data: Configure Magnet Type" {
        # "Do not put any code in this frame.\n(It is a separator no-op. You can make a copy of this frame to create a new Data frame)"
        n103 = Unbundle By Name(w256) -> ("Instruments.Magnet"=w261:refnum<class "Instrument.Cryostat.lvclass">)
        n104 = call <vilib>:"Get LV Class Name.vi"("error in (no error)"=w265, "object"=w261) -> ("error out"=w259:errorcluster, "class name"=w269:string)  [unwired: 8 in]
        n105 = Match Pattern(string=w269, regular expression="VRM") -> (offset past match=w267:i32)  [unwired: 1 in, 3 out]
        n106 = Greater Or Equal To 0?(x=w267) -> (x >= 0?=w257:bool)
        n107 = Select(t="Vector Magnet" ("new element/subarray"), s=w257, f="Magnet" ("element")) -> (s? t:f=w262:string)
        n108 = call "Set StateName.vi"("error in (no error)"=w259, "StateName"=w262, "SMO"=w261) -> ("error out"=w258:errorcluster, "SMO out"=w260:refnum<class "Instrument.Cryostat.lvclass">)  [unwired: 7 in]
        n109 = Bundle By Name(cluster=w256, "Instruments.Magnet"=w260) -> (w266:T14)
        n110 = call <vilib>:"Add State(s) to Queue__jki_lib_state_machine.vi"("State(s) in (\"\")"=w271) -> ("States Out"=w270:string)  [unwired: 14 in]
      }
      frame "Data: Close Instruments" {
        # "Data: Close Instruments\n(Close Instruments that are explicitly opened by this VI)"
        n111 = Unbundle By Name(w277) -> ("Instruments"=w274:T13)
        n112 = call <vilib>:"Get Cluster Information.vi"("variant"=w274) -> ("error out"=w272:errorcluster, "cluster elements"=w273:variant[])  [unwired: 9 in]
        n113 = Cluster To Array(cluster=w274) -> (array=w280:refnum<class "Instrument.lvclass">[])
        n114 = for {
          tunnel: w280 -> [w287] mode=indexing
          tunnel: [w293] -> w281 mode=indexing
          shift-right: [w296] -> w279
          shift-left: w274 -> [w297]
          tunnel: w273 -> [w290] mode=indexing
          tunnel: w272 -> [w288]
          n115 = call <vilib>:"Get Type Information.vi"("error in (no error)"=w288, "variant"=w290) -> ("name"=w289:string)  [unwired: 5 in, 4 out]
          n116 = call "Get IsConfigured.vi"("SMO"=w287) -> ("error out"=w284:errorcluster, "IsConfigured?"=w286:bool, "SMO out"=w285:refnum<class "Instrument.lvclass">)  [unwired: 8 in]
          n117 = case shown="True" w286 {
            tunnel: [w298 w302] -> w294
            tunnel: w285 -> [w299 w301]
            tunnel: [w299 w300] -> w295
            tunnel: w284 -> [w298 _]
            frame False {
            }
            frame True {
              n118 = call-dynamic "Close.vi"("Instrument in"=w301) -> ("error out"=w302:errorcluster, "Instrument out"=w300:refnum<class "Instrument.lvclass">)  [unwired: 9 in]
            }
          }
          n119 = Scan From String(input string=w289, default 1=Instrument_Types--enum."DAQ" ("Type")) -> (output 1=w291:T8)  [unwired: 3 in, 3 out]
          n120 = call "Cast Instrument to Instrument Type.vi"("error in (no error)"=w294, "Type"=w291, "Instrument in"=w295, "Instrument Classes"=w297) -> ("error out"=w293:errorcluster, "Instrument Classes out"=w296:T13)  [unwired: 5 in, 1 out]
        }
        n121 = Bundle By Name(cluster=w277, "Instruments"=w279) -> (w276:T14)
        n122 = Merge Errors(w278, w281) -> (w275:errorcluster)
        n123 = call <vilib>:"Add State(s) to Queue__jki_lib_state_machine.vi"("State(s) in (\"\")"=w283) -> ("States Out"=w282:string)  [unwired: 14 in]
      }
      frame "Data: UI Stop" {
        # "Data: UI Stop\n(Used to record when stop signal comes from UI (front panel stop or panel close)"
        n124 = Scan From String(input string=w305, default 1=FALSE) -> (output 1=w304:bool)  [unwired: 3 in, 3 out]
        n125 = Bundle By Name(cluster=w306, "UI stop"=w304) -> (w307:T14)
        n126 = call <vilib>:"Add State(s) to Queue__jki_lib_state_machine.vi"("State(s) in (\"\")"=w310) -> ("States Out"=w309:string)  [unwired: 14 in]
      }
      frame "Data: Cleanup" {
        # "Cleanup any data and references, here.\n(this is called automatically, by the Macro: Exit)"
        n127 = Unbundle By Name(w325) -> ("Transport"=w329:refnum<class "Transport.lvclass">, "Execution:State"=w322:T7, "C.E."=w321:refnum<class "Control Experiment.lvclass">, "Instruments"=w320:T13, "Core.Current VI Reference"=w327:refnum<vi>)
        n128 = case shown="\"Run top level\"" w322 {
          tunnel: [w334 w339] -> w319
          tunnel: w321 -> [w334 w338]
          tunnel: w317 -> [w332 w336]
          tunnel: [w332 w337] -> w316
          tunnel: w320 -> [w333 w335]
          tunnel: [w333 w335] -> w318
          frame Default {
          }
          frame "Run top level" {
            n129 = call "Close Dictionary.vi"("error in (no error)"=w336, "Control Experiment in"=w338) -> ("error out"=w337:errorcluster, "Control Experiment out"=w339:refnum<class "Control Experiment.lvclass">)  [unwired: 8 in]
          }
        }
        n130 = call "Write Instruments.vi"("error in (no error)"=w316, "Instruments"=w318, "Control Experiment in"=w319) -> ("error out"=w323:errorcluster, "Control Experiment out"=w324:refnum<class "Control Experiment.lvclass">)  [unwired: 7 in]
        n131 = call "Write Dependencies.vi"("error in (no error)"=w323, "Control Experiment"=w324, "Transport in"=w329) -> ("error out"=w312:errorcluster, "Transport out"=w314:refnum<class "Transport.lvclass">)  [unwired: 7 in]
        n132 = call "Send RunningStatus Notifier.vi"("error in (no error)"=w312, "Running?"=FALSE, "Transport in"=w314) -> ("error out"=w311:errorcluster, "Transport out"=w313:refnum<class "Transport.lvclass">)  [unwired: 7 in]
        n133 = Bundle By Name(cluster=w325, "Transport"=w313) -> (w328:T14)
        n134 = Close Reference(reference=w327, error in (no error)=w311) -> (error out=w326:errorcluster)
        n135 = call <vilib>:"Add State(s) to Queue__jki_lib_state_machine.vi"("State(s) in (\"\")"=w331) -> ("States Out"=w330:string)  [unwired: 14 in]
      }
      frame "---------- UI ----------" {
        # "Do not put any code in this frame.\n(It is a separator no-op. You can make a copy of this frame to create a new UI frame)"
        n136 = call <vilib>:"Add State(s) to Queue__jki_lib_state_machine.vi"("State(s) in (\"\")"=w343) -> ("States Out"=w342:string)  [unwired: 14 in]
      }
      frame "UI: Initialize" {
        # "Initialize the User Interface, here.\n(this is called automatically, by the Macro: Init)"
        n137 = call <userlib>:"Tick Count (ms)__ogtk.vi"("error in (no error)"=w351) -> ("error out"=w350:errorcluster, "millisecond timer value"=w349:u32)  [unwired: 9 in]
        n138 = call <userlib>:"Fit VI window to Largest Dec__ogtk.vi"("error in (no error)"=w350, "border spacing (2 px)"=0) -> ("error out"=w346:errorcluster)  [unwired: 4 in, 1 out]
        n139 = local read "Emergency Stop Visible?"() -> (w345:bool)
        n140 = invoke on="stop" class="Bool (strict)" method="Reinit To Default"() -> ()  [unwired: 3 in, 3 out]
        n141 = property on="Emergency Stop Visible?" class="Bool (strict)"("Val(Sgnl)"=w345) -> ()  [unwired: 2 in, 2 out]
        n142 = Bundle By Name(cluster=w344, "ms [0]"=w349, "ms [i]"=w349) -> (w347:T14)
        n143 = call <vilib>:"Add State(s) to Queue__jki_lib_state_machine.vi"("State(s) in (\"\")"=w353) -> ("States Out"=w352:string)  [unwired: 14 in]
      }
      frame "UI: Cursor Set" {
        # "Argument"
        # "Set and Unset Cursor Busy.\n(Usage: \"UI: Cursor Set >> Busy|Idle\")"
        n144 = case shown="\"Idle\", Default" w354 {
          tunnel: w356 -> [w361 w363]
          tunnel: [w360 w362] -> w355
          frame "Idle", Default {
            n145 = call <vilib>:"Unset Busy.vi"("error in (no error)"=w361) -> ("error out"=w360:errorcluster)  [unwired: 10 in]
          }
          frame "Busy" {
            n146 = call <vilib>:"Set Busy.vi"("error in (no error)"=w363) -> ("error out"=w362:errorcluster)  [unwired: 9 in, 1 out]
          }
        }
        n147 = call <vilib>:"Add State(s) to Queue__jki_lib_state_machine.vi"("State(s) in (\"\")"=w359) -> ("States Out"=w358:string)  [unwired: 14 in]
      }
      frame "UI: Emergency Stop Visible" {
        # "Do not put any code in this frame.\n(It is a separator no-op. You can make a copy of this frame to create a new UI frame)"
        n148 = Scan From String(input string=w366, default 1=FALSE) -> (output 1=w364:bool)  [unwired: 3 in, 3 out]
        n149 = property on="Emergency Stop 1" class="Bool"("Visible"=w364) -> ()  [unwired: 2 in, 2 out]
        n150 = property on="Emergency Stop 2" class="Bool"("Visible"=w364) -> ()  [unwired: 2 in, 2 out]
        n151 = property on="Emergency Stop 3" class="Bool"("Visible"=w364) -> ()  [unwired: 2 in, 2 out]
        n152 = property on="Emergency Stop 4" class="Bool"("Visible"=w364) -> ()  [unwired: 2 in, 2 out]
        n153 = call <vilib>:"Add State(s) to Queue__jki_lib_state_machine.vi"("State(s) in (\"\")"=w370) -> ("States Out"=w369:string)  [unwired: 14 in]
      }
      frame "UI: Update Timer" {
        n154 = Unbundle By Name(w382) -> ("ms [0]"=w383:u32)
        n155 = call <userlib>:"Tick Count (ms)__ogtk.vi"("error in (no error)"=w373) -> ("error out"=w372:errorcluster, "millisecond timer value"=w377:u32)  [unwired: 9 in]
        n156 = Subtract(x=w377, y=w383) -> (x-y=w380:u32)
        n157 = call <userlib>:"MGI Milliseconds Since Last Call.vi"("Error In"=w372) -> ("ms"=→"time b/w points (ms)":u32, "Error Out"=w378:errorcluster)  [unwired: 5 in]
        n158 = To Double Precision Float(number=w380) -> (double precision float=w376:dbl)
        n159 = To Double Precision Float(number=u32 1000 ("x")) -> (double precision float=w375:dbl)
        n160 = Bundle By Name(cluster=w382, "ms [i]"=w377) -> (w381:T14)
        n161 = Divide(x=w376, y=w375) -> (x/y=w384:dbl)
        n162 = To Long Integer(number=w384) -> (32bit integer=→"elapsed time (s)":i32)
        n163 = call <vilib>:"Add State(s) to Queue__jki_lib_state_machine.vi"("State(s) in (\"\")"=w386) -> ("States Out"=w385:string)  [unwired: 14 in]
      }
      frame "UI: Update Status" {
        # "Do not put any code in this frame.\n(It is a separator no-op. You can make a copy of this frame to create a new UI frame)"
        n164 = local read "Instrument Status"() -> (w389:string)
        n165 = To Lower Case(string=w388) -> (all lower case string=w396:string)
        n166 = Empty String/Path?(string/path=w389) -> (empty?=w387:bool)
        n167 = Equal?(x=w396, y="reset") -> (x = y?=w395:bool)
        n168 = Format Into String(format string="%s, %s", w389, w388) -> (resulting string=w391:string)  [unwired: 2 in, 1 out]
        n169 = Select(t=w388, s=w387, f=w391) -> (s? t:f=w390:string)
        n170 = Select(t="", s=w395, f=w390) -> (s? t:f=→"Instrument Status":string)
        n171 = call <vilib>:"Add State(s) to Queue__jki_lib_state_machine.vi"("State(s) in (\"\")"=w401) -> ("States Out"=w400:string)  [unwired: 14 in]
      }
      frame "UI: Update Graph Axis Labels" {
        w404 = "sweep (V)" ("string")
        n172 = control-ref of="AO"() -> (w406:refnum<vi>)
        n173 = control-ref of="AI"() -> (w405:refnum<vi>)
        n174 = control-ref of="2 Terminal"() -> (w410:refnum<vi>)
        n175 = control-ref of="4 Terminal"() -> (w409:refnum<vi>)
        n176 = control-ref of="Lockin (X)"() -> (w419:refnum<vi>)
        n177 = control-ref of="Lockin (Y)"() -> (w418:refnum<vi>)
        n178 = control-ref of="Resistance"() -> (w416:refnum<vi>)
        n179 = control-ref of="Conductance"() -> (w411:refnum<vi>)
        n180 = local read "Units"() -> (w414:enum16{"ohms & siemens", "h/e2 & e2/h"})
        n181 = case shown="\"h/e2 & e2/h\"" w414 {
          tunnel: ["R (ohms)" "R (h/e2)"] -> w413
          tunnel: ["G (siemens)" "G (e2/h)"] -> w412
          frame "ohms & siemens", Default {
          }
          frame "h/e2 & e2/h" {
          }
        }
        n182 = property on="Property Node" class="XYGraph (strict)"(reference=w410, "XScale.NameLbl.Text"=w404) -> (error out=w407:errorcluster)  [unwired: 1 in, 1 out]
        n183 = property on="Property Node" class="XYGraph (strict)"(reference=w409, "XScale.NameLbl.Text"=w404) -> (error out=w408:errorcluster)  [unwired: 1 in, 1 out]
        n184 = property on="Property Node" class="XYGraph (strict)"(reference=w419, "XScale.NameLbl.Text"=w404) -> (error out=w423:errorcluster)  [unwired: 1 in, 1 out]
        n185 = property on="Property Node" class="XYGraph (strict)"(reference=w418, "XScale.NameLbl.Text"=w404) -> (error out=w424:errorcluster)  [unwired: 1 in, 1 out]
        n186 = property on="Property Node" class="XYGraph (strict)"(reference=w416, "XScale.NameLbl.Text"=w404, "YScale.NameLbl.Text"=w413) -> (error out=w425:errorcluster)  [unwired: 1 in, 1 out]
        n187 = property on="Property Node" class="XYGraph (strict)"(reference=w411, "XScale.NameLbl.Text"=w404, "YScale.NameLbl.Text"=w412) -> (error out=w415:errorcluster)  [unwired: 1 in, 1 out]
        n188 = property on="Property Node" class="XYGraph (strict)"(reference=w406, "XScale.NameLbl.Text"=w404) -> (error out=w402:errorcluster)  [unwired: 1 in, 1 out]
        n189 = property on="Property Node" class="XYGraph (strict)"(reference=w405, "XScale.NameLbl.Text"=w404) -> (error out=w403:errorcluster)  [unwired: 1 in, 1 out]
        n190 = Merge Errors(w402, w403, w407, w408, w423, w424, w425, w415, w421) -> (w420:errorcluster)
        n191 = call <vilib>:"Clear Errors.vi"("error in (no error)"=w420) -> ("error out"=w422:errorcluster)  [unwired: 5 in, 1 out]
        n192 = call <vilib>:"Add State(s) to Queue__jki_lib_state_machine.vi"("State(s) in (\"\")"=w427) -> ("States Out"=w426:string)  [unwired: 14 in]
      }
      frame "UI: Update Lockin Graph Legend" {
        n193 = Unbundle By Name(w440) -> ("Results (Dictionary)"=w437:cluster{"key":string, "value":dbl}[])
        n194 = call <userlib>:"Parse Results (all).vi"("Type"=Results_Type--Enum."X", "error in (no error)"=w438, "Results (Dictionary)"=w437) -> ("error out"=w439:errorcluster, "Label"=w434:string[])  [unwired: 5 in, 2 out]
        n195 = Array Size(array=w434) -> (size(s)=w435:i32)
        n196 = for {
          tunnel: w439 -> [w452]
          tunnel: w434 -> [w448] mode=indexing
          tunnel: w435 -> [w447]
          tunnel: [w446] -> w433 mode=indexing
          tunnel: [w445] -> w432 mode=indexing
          i -> [w451]
          n197 = control-ref of="Lockin (X)"() -> (w449:refnum<vi>)
          n198 = property on="Property Node" class="XYGraph (strict)"(reference=w449, error in=w452, "Active Plot"=w451, "Plot.Plot Name"=w448, "LegPlotMin"=w447) -> (error out=w445:errorcluster)  [unwired: 1 out]
          n199 = control-ref of="Lockin (Y)"() -> (w450:refnum<vi>)
          n200 = property on="Property Node" class="XYGraph (strict)"(reference=w450, "Active Plot"=w451, "Plot.Plot Name"=w448, "LegPlotMin"=w447) -> (error out=w446:errorcluster)  [unwired: 1 in, 1 out]
        }
        n201 = Merge Errors(w433, w432) -> (w436:errorcluster)
        n202 = call <vilib>:"Clear Errors.vi"("error in (no error)"=w436) -> ("error out"=w442:errorcluster)  [unwired: 5 in, 1 out]
        n203 = call <vilib>:"Add State(s) to Queue__jki_lib_state_machine.vi"("State(s) in (\"\")"=w444) -> ("States Out"=w443:string)  [unwired: 14 in]
      }
      frame "UI: Update Wfm Graph Legend" {
        n204 = Unbundle By Name(w461) -> ("AO Waveforrm"=w458:waveform(dbl)[], "AI Waveform"=w457:waveform(dbl)[])
        n205 = Array Size(array=w457) -> (size(s)=w456:i32)
        n206 = Array Size(array=w458) -> (size(s)=w459:i32)
        n207 = for {
          N: w459 -> [w472]
          tunnel: [w477] -> w454 mode=indexing
          i -> [w476]
          n208 = Increment(x=w476) -> (x+1=w473:i32)
          n209 = control-ref of="AO"() -> (w478:refnum<vi>)
          n210 = Format Into String(format string="AO %d", w473) -> (resulting string=w474:string)  [unwired: 2 in, 1 out]
          n211 = property on="Property Node" class="XYGraph (strict)"(reference=w478, "Active Plot"=w476, "Plot.Plot Name"=w474, "LegPlotMin"=w472) -> (error out=w477:errorcluster)  [unwired: 1 in, 1 out]
        }
        n212 = for {
          N: w456 -> [w466]
          tunnel: [w471] -> w455 mode=indexing
          i -> [w470]
          n213 = Increment(x=w470) -> (x+1=w467:i32)
          n214 = control-ref of="AI"() -> (w465:refnum<vi>)
          n215 = Format Into String(format string="AI %d", w467) -> (resulting string=w468:string)  [unwired: 2 in, 1 out]
          n216 = property on="Property Node" class="XYGraph (strict)"(reference=w465, "Active Plot"=w470, "Plot.Plot Name"=w468, "LegPlotMin"=w466) -> (error out=w471:errorcluster)  [unwired: 1 in, 1 out]
        }
        n217 = Merge Errors(w454, w455, w453) -> (w460:errorcluster)
        n218 = call <vilib>:"Clear Errors.vi"("error in (no error)"=w460) -> ("error out"=w462:errorcluster)  [unwired: 5 in, 1 out]
        n219 = call <vilib>:"Add State(s) to Queue__jki_lib_state_machine.vi"("State(s) in (\"\")"=w464) -> ("States Out"=w463:string)  [unwired: 14 in]
      }
      frame "UI: Update R G Graph Legend" {
        n220 = local read "Resistance"() -> (w494:cluster{"X-array":dbl[], "Y-array":dbl[]}[])
        n221 = local read "Conductance"() -> (w495:cluster{"X-array":dbl[], "Y-array":dbl[]}[])
        n222 = Array Size(array=w494) -> (size(s)=w483:i32)
        n223 = Array Size(array=w495) -> (size(s)=w493:i32)
        n224 = Quotient & Remainder(x=w483, y=2) -> (floor(x/y)=w480:i32)  [unwired: 1 out]
        n225 = Quotient & Remainder(x=w493, y=2) -> (floor(x/y)=w487:i32)  [unwired: 1 out]
        n226 = Greater?(x=w480, y=1) -> (0:w479:bool)
        n227 = Greater?(x=w487, y=1) -> (0:w490:bool)
        n228 = case shown="True" w479 {
          tunnel: string[] ["R2T", "R4T"] -> [w503 w506]
          tunnel: [w503 w504] -> w482
          tunnel: w480 -> [_ w505]
          frame False {
          }
          frame True {
            n229 = for {
              N: w505 -> [_]
              tunnel: w506 -> [w509]
              tunnel: [w507] -> w504 mode=concatenating
              i -> [w511]
              n230 = call <vilib>:"Space Constant.vi"() -> ("String"=w510:string)
              n231 = Format Into String(initial string=w510, w511) -> (resulting string=w508:string)  [unwired: 2 in, 1 out]
              n232 = for {
                tunnel: w509 -> [w514] mode=indexing
                tunnel: w508 -> [w513]
                tunnel: [w512] -> w507 mode=indexing
                n233 = Concatenate Strings(w514, w513) -> (w512:string)
              }
            }
          }
        }
        n234 = case shown="False" w490 {
          tunnel: string[] ["G2T", "G4T"] -> [w515 w518]
          tunnel: [w515 w516] -> w491
          tunnel: w487 -> [_ w517]
          frame False {
          }
          frame True {
            n235 = for {
              N: w517 -> [_]
              tunnel: w518 -> [w521]
              tunnel: [w519] -> w516 mode=concatenating
              i -> [w523]
              n236 = call <vilib>:"Space Constant.vi"() -> ("String"=w522:string)
              n237 = Format Into String(initial string=w522, w523) -> (resulting string=w520:string)  [unwired: 2 in, 1 out]
              n238 = for {
                tunnel: w521 -> [w526] mode=indexing
                tunnel: w520 -> [w525]
                tunnel: [w524] -> w519 mode=indexing
                n239 = Concatenate Strings(w526, w525) -> (w524:string)
              }
            }
          }
        }
        n240 = for {
          N: w493 -> [w534]
          tunnel: [w535] -> w496 mode=indexing
          tunnel: w491 -> [w532] mode=indexing
          i -> [w533]
          n241 = control-ref of="Conductance"() -> (w536:refnum<vi>)
          n242 = property on="Property Node" class="XYGraph (strict)"(reference=w536, "Active Plot"=w533, "Plot.Plot Name"=w532, "LegPlotMin"=w534) -> (error out=w535:errorcluster)  [unwired: 1 in, 1 out]
        }
        n243 = for {
          N: w483 -> [w529]
          tunnel: [w531] -> w497 mode=indexing
          tunnel: w482 -> [w527] mode=indexing
          i -> [w530]
          n244 = control-ref of="Resistance"() -> (w528:refnum<vi>)
          n245 = property on="Property Node" class="XYGraph (strict)"(reference=w528, "Active Plot"=w530, "Plot.Plot Name"=w527, "LegPlotMin"=w529) -> (error out=w531:errorcluster)  [unwired: 1 in, 1 out]
        }
        n246 = Merge Errors(w496, w497, w486) -> (w498:errorcluster)
        n247 = call <vilib>:"Add State(s) to Queue__jki_lib_state_machine.vi"("State(s) in (\"\")"=w502) -> ("States Out"=w501:string)  [unwired: 14 in]
        n248 = call <vilib>:"Clear Errors.vi"("error in (no error)"=w498) -> ("error out"=w500:errorcluster)  [unwired: 5 in, 1 out]
      }
      frame "UI: Update AO AI Graphs" {
        n249 = Unbundle By Name(w549) -> ("Sweep Value"=w537:dbl, "AO Waveforrm"=w543:waveform(dbl)[], "AI Waveform"=w544:waveform(dbl)[])  [unwired: 1 out]
        n250 = To Lower Case(string=w545) -> (all lower case string=w546:string)
        n251 = Equal?(x=w546, y="reset") -> (x = y?=w540:bool)
        n252 = for {
          tunnel: w543 -> [w553] mode=indexing
          tunnel: [w552] -> w539 mode=indexing
          n253 = Unbundle By Name(w553) -> ("Y"=w554:dbl[])
          n254 = Index Array(array=w554) -> (element=w552:dbl)  [unwired: 1 in]
        }
        n255 = for {
          tunnel: w544 -> [w556] mode=indexing
          tunnel: [w555] -> w538 mode=indexing
          n256 = Unbundle By Name(w556) -> ("Y"=w557:dbl[])
          n257 = Index Array(array=w557) -> (element=w555:dbl)  [unwired: 1 in]
        }
        n258 = call "Graph Lockin vs Parameter.vi"("reset?"=w540, "Y"=w539, "X"=w537) -> ("Data vs Parameter"=→"AO":cluster{dbl[], dbl[]}[])  [unwired: 8 in]
        n259 = call "Graph Lockin vs Parameter.vi"("reset?"=w540, "Y"=w538, "X"=w537) -> ("Data vs Parameter"=→"AI":cluster{dbl[], dbl[]}[])  [unwired: 8 in]
        n260 = call <vilib>:"Add State(s) to Queue__jki_lib_state_machine.vi"("State(s) in (\"\")"=w551) -> ("States Out"=w550:string)  [unwired: 14 in]
      }
      frame "UI: Update Lockin Graphs" {
        # "results"
        n261 = Unbundle By Name(w568) -> ("Sweep Value"=w558:dbl, "Results (Dictionary)"=w574:cluster{"key":string, "value":dbl}[])  [unwired: 1 out]
        n262 = To Lower Case(string=w565) -> (all lower case string=w566:string)
        n263 = Equal?(x=w566, y="reset") -> (x = y?=w559:bool)
        n264 = call <userlib>:"Parse Results (all).vi"("Type"=Results_Type--Enum."X", "error in (no error)"=w563, "Results (Dictionary)"=w574) -> ("error out"=w570:errorcluster, "Data"=w561:dbl[], "Results (Dictionary)"=w571:cluster{"key":string, "value":dbl}[])  [unwired: 5 in, 1 out]
        n265 = call <userlib>:"Parse Results (all).vi"("Type"=Results_Type--Enum."Y", "error in (no error)"=w570, "Results (Dictionary)"=w571) -> ("error out"=w569:errorcluster, "Data"=w560:dbl[])  [unwired: 5 in, 2 out]
        n266 = call "Graph Lockin vs Parameter.vi"("reset?"=w559, "Y"=w561, "X"=w558) -> ("Data vs Parameter"=→"Lockin (X)":cluster{dbl[], dbl[]}[])  [unwired: 8 in]
        n267 = call "Graph Lockin vs Parameter.vi"("reset?"=w559, "Y"=w560, "X"=w558) -> ("Data vs Parameter"=→"Lockin (Y)":cluster{dbl[], dbl[]}[])  [unwired: 8 in]
        n268 = call <vilib>:"Add State(s) to Queue__jki_lib_state_machine.vi"("State(s) in (\"\")"=w576) -> ("States Out"=w575:string)  [unwired: 14 in]
      }
      frame "UI: Update R G Graphs" {
        # "Do not put any code in this frame.\n(It is a separator no-op. You can make a copy of this frame to create a new UI frame)"
        n269 = Unbundle By Name(w583) -> ("Amplitude"=w582:dbl[], "C.E."=w581:refnum<class "Control Experiment.lvclass">)
        n270 = call "Get Channel Indices.vi"("Control Experiment in"=w581) -> ("Indices"=w580:T16)  [unwired: 8 in, 2 out]
        n271 = local read "Lockin (Y)"() -> (w584:cluster{"Wavenumber":dbl[], "Data":dbl[]}[])
        n272 = local read "Lockin (X)"() -> (w585:cluster{"Wavenumber":dbl[], "Data":dbl[]}[])
        n273 = case shown="\"h/e2 & e2/h\"" "Units" {
          tunnel: [1.0 ("Siemens/(e2/h)") w593] -> w588
          frame "ohms & siemens", Default {
          }
          frame "h/e2 & e2/h" {
            w593 = 3.874046e-05  # Siemens/(e2/h)
          }
        }
        n274 = call "Graph R and G vs Parameter.vi"("indices"=w580, "AO Amp (V)"=w582, "Y vs Parameter"=w584, "X vs Parameter"=w585) -> ("G(Siemens) vs Parameter"=w587:cluster{"X-array":dbl[], dbl[]}[], "R(Ohms) vs Parameter"=w586:cluster{"X-array":dbl[], dbl[]}[])  [unwired: 6 in]
        n275 = call-poly <vilib>:"Multiply.vi"("y (1)"=w588, "XY-data"=w586) -> ("XY-data out"=→"Resistance":cluster{"X-array":dbl[], "Y-array":dbl[]}[])  [unwired: 8 in, 1 out]
        n276 = call-poly <vilib>:"Divide.vi"("y (1)"=w588, "XY-data"=w587) -> ("XY-data out"=→"Conductance":cluster{"X-array":dbl[], "Y-array":dbl[]}[])  [unwired: 8 in, 1 out]
        n277 = call <vilib>:"Add State(s) to Queue__jki_lib_state_machine.vi"("State(s) in (\"\")"=w591) -> ("States Out"=w590:string)  [unwired: 14 in]
      }
      frame "UI: Update Graphs from wfm" {
        # "Do not put any code in this frame.\n(It is a separator no-op. You can make a copy of this frame to create a new UI frame)"
        n278 = local read "Sweep Channels"() -> (w604:T2)
        n279 = Unbundle By Name(w606) -> ("Sweep_AO"=w601:waveform(dbl)[], "Sweep_AI"=w600:waveform(dbl)[], "Sweep_X"=w599:waveform(dbl)[], "Sweep_Y"=w598:waveform(dbl)[])  [unwired: 1 out]
        n280 = for {
          tunnel: [w622] -> w603
          tunnel: w604 -> [w625] mode=indexing
          stop <- w624 stop-if-true
          # "find the 1st enabled channel"
          n281 = Unbundle By Name(w625) -> ("Enable?"=w624:bool, "Channel"=w623:u16)
          n282 = Decrement(x=w623) -> (x-1=w622:u16)
        }
        n283 = Index Array(array=w601, index=w603) -> (element=w605:waveform(dbl))
        n284 = Unbundle By Name(w605) -> ("Y"=w597:dbl[])
        n285 = for {
          tunnel: w597 -> [w618]
          tunnel: w600 -> [w620] mode=indexing
          tunnel: [w619] -> w594 mode=indexing
          n286 = Unbundle By Name(w620) -> ("Y"=w621:dbl[])
          n287 = call <vilib>:"Initialize.vi"("Y-array"=w621, "X-array"=w618) -> ("XY-data out"=w619:cluster{"X-array":dbl[], "Y-array":dbl[]})  [unwired: 8 in, 1 out]
        }
        n288 = for {
          tunnel: w597 -> [w626]
          tunnel: w601 -> [w628] mode=indexing
          tunnel: [w627] -> w602 mode=indexing
          n289 = Unbundle By Name(w628) -> ("Y"=w629:dbl[])
          n290 = call <vilib>:"Initialize.vi"("Y-array"=w629, "X-array"=w626) -> ("XY-data out"=w627:cluster{"X-array":dbl[], "Y-array":dbl[]})  [unwired: 8 in, 1 out]
        }
        n291 = for {
          tunnel: w597 -> [w610]
          tunnel: w598 -> [w612] mode=indexing
          tunnel: [w611] -> w596 mode=indexing
          n292 = Unbundle By Name(w612) -> ("Y"=w613:dbl[])
          n293 = call <vilib>:"Initialize.vi"("Y-array"=w613, "X-array"=w610) -> ("XY-data out"=w611:cluster{"X-array":dbl[], "Y-array":dbl[]})  [unwired: 8 in, 1 out]
        }
        n294 = for {
          tunnel: w597 -> [w614]
          tunnel: w599 -> [w616] mode=indexing
          tunnel: [w615] -> w595 mode=indexing
          n295 = Unbundle By Name(w616) -> ("Y"=w617:dbl[])
          n296 = call <vilib>:"Initialize.vi"("Y-array"=w617, "X-array"=w614) -> ("XY-data out"=w615:cluster{"X-array":dbl[], "Y-array":dbl[]})  [unwired: 8 in, 1 out]
        }
        n297 = local write "AO"(w602) -> ()
        n298 = local write "AI"(w594) -> ()
        n299 = local write "Lockin (X)"(w595) -> ()
        n300 = local write "Lockin (Y)"(w596) -> ()
        n301 = call <vilib>:"Add State(s) to Queue__jki_lib_state_machine.vi"("State(s) in (\"\")"=w609) -> ("States Out"=w608:string)  [unwired: 14 in]
      }
      frame "UI: Update IV Graphs" {
        # "Do not put any code in this frame.\n(It is a separator no-op. You can make a copy of this frame to create a new UI frame)"
        n302 = Unbundle By Name(w646) -> ("Sweep_AI"=w643:waveform(dbl)[], "Sweep_AO"=w642:waveform(dbl)[], "C.E."=w648:refnum<class "Control Experiment.lvclass">)
        n303 = call "Get Channel Indices.vi"("error in (no error)"=w638, "Control Experiment in"=w648) -> ("error out"=w637:errorcluster, "Indices"=w635:T16)  [unwired: 7 in, 1 out]
        n304 = Decrement(x=w635) -> (x-1=w634:T16)
        n305 = Unbundle By Name(w634) -> ("I-"=w649:i32, "V1+"=w647:i32, "V1-"=w633:i32, "I+"=w652:i32)
        n306 = Equal?(x=w647, y=w633) -> (x = y?=w631:bool)
        n307 = Index Array(array=w643, index #1=w649, index #2=w647, index #3=w633) -> (element #1=w636:waveform(dbl), element #2=w651:waveform(dbl), element #3=w632:waveform(dbl))
        n308 = Index Array(array=w642, index=w652) -> (element=w653:waveform(dbl))
        n309 = case shown="False" w631 {
          tunnel: w651 -> [w657 w661]
          tunnel: w632 -> [_ w660]
          tunnel: [w657 w659] -> w630
          tunnel: [_ w658] -> _
          frame True {
          }
          frame False {
            n310 = Subtract(1:w660, 2:w661) -> (0:w659:waveform(dbl), 3:w658:errorcluster)  [unwired: 1 in]
          }
        }
        n311 = Unbundle By Name(w636) -> ("Y"=w641:dbl[])
        n312 = Unbundle By Name(w630) -> ("Y"=w640:dbl[])
        n313 = Unbundle By Name(w653) -> ("Y"=w639:dbl[])
        n314 = Bundle("Y"=w640, "Y"=w641) -> (w650:cluster{"Y":dbl[], "Y":dbl[]})  [unwired: 1 in]
        n315 = Bundle("Y"=w639, "Y"=w641) -> (w654:cluster{"Y":dbl[], "Y":dbl[]})  [unwired: 1 in]
        n316 = Build Array(w650) -> (→"4 Terminal":cluster{"Y":dbl[], "Y":dbl[]}[])
        n317 = Build Array(w654) -> (→"2 Terminal":cluster{"Y":dbl[], "Y":dbl[]}[])
        n318 = call <vilib>:"Add State(s) to Queue__jki_lib_state_machine.vi"("State(s) in (\"\")"=w656) -> ("States Out"=w655:string)  [unwired: 14 in]
      }
      frame "UI: Front Panel State" {
        # "Argument"
        # "Set Front Panel Open or Closed\n(Usage: \"UI: Front Panel State >> Open|Close\")"
        n319 = Unbundle By Name(w664) -> ("Core.Current VI Reference"=w663:refnum<vi>)
        n320 = case shown="\"Maximize\", \"Maximized\"" w662 {
          tunnel: w666 -> [w674 w689 w700 w713 w726]
          tunnel: [w676 w690 w702 w715 w728] -> w665
          tunnel: w663 -> [w675 w687 w701 w714 w727]
          frame "Open", "Standard", Default {
            w669 = T5."Standard" ("State")
            n321 = property class="VI"(reference=w675, error in=w674) -> (reference out=w672:refnum<vi>, error out=w673:errorcluster, "FP.State"=w671:T5)
            n322 = Not Equal?(x=w671, y=w669) -> (x != y?=w670:bool)
            n323 = case shown="False" w670 {
              tunnel: [w680 w682] -> w676
              tunnel: w673 -> [w679 w682]
              tunnel: w672 -> [w678 _]
              tunnel: w669 -> [w677 _]
              frame True {
                n324 = invoke class="VI" method="FP.Open"(reference=w678, error in=w679, "Activate"=TRUE, "State"=w677) -> (error out=w680:errorcluster)  [unwired: 1 in, 4 out]
              }
              frame False {
              }
            }
          }
          frame "Close", "Closed" {
            n325 = property class="VI"(reference=w687, error in=w689) -> (reference out=w686:refnum<vi>, error out=w688:errorcluster, "FP.State"=w684:T5)
            n326 = Not Equal?(x=w684, y=T5."Closed" ("Front Panel Window:State")) -> (x != y?=w683:bool)
            n327 = case shown="True" w683 {
              tunnel: [w691 w694] -> w690
              tunnel: w688 -> [w691 w693]
              tunnel: w686 -> [_ w692]
              frame False {
              }
              frame True {
                n328 = invoke class="VI" method="FP.Close"(reference=w692, error in=w693) -> (error out=w694:errorcluster)  [unwired: 1 in, 2 out]
              }
            }
          }
          frame "Hidden", "Hide" {
            w695 = T5."Hidden" ("State")
            n329 = property class="VI"(reference=w701, error in=w700) -> (reference out=w698:refnum<vi>, error out=w699:errorcluster, "FP.State"=w697:T5)
            n330 = Not Equal?(x=w697, y=w695) -> (x != y?=w696:bool)
            n331 = case shown="True" w696 {
              tunnel: [w706 w707] -> w702
              tunnel: w699 -> [w705 w707]
              tunnel: w698 -> [w704 _]
              tunnel: w695 -> [w703 _]
              frame True {
                n332 = invoke class="VI" method="FP.Open"(reference=w704, error in=w705, "State"=w703) -> (error out=w706:errorcluster)  [unwired: 2 in, 4 out]
              }
              frame False {
              }
            }
          }
          frame "Minimize", "Minimized" {
            w708 = T5."Minimized" ("State")
            n333 = property class="VI"(reference=w714, error in=w713) -> (reference out=w711:refnum<vi>, error out=w712:errorcluster, "FP.State"=w710:T5)
            n334 = Not Equal?(x=w710, y=w708) -> (x != y?=w709:bool)
            n335 = case shown="True" w709 {
              tunnel: [w719 w720] -> w715
              tunnel: w712 -> [w718 w720]
              tunnel: w711 -> [w717 _]
              tunnel: w708 -> [w716 _]
              frame True {
                n336 = invoke class="VI" method="FP.Open"(reference=w717, error in=w718, "State"=w716) -> (error out=w719:errorcluster)  [unwired: 2 in, 4 out]
              }
              frame False {
              }
            }
          }
          frame "Maximize", "Maximized" {
            w721 = T5."Maximized" ("State")
            n337 = property class="VI"(reference=w727, error in=w726) -> (reference out=w724:refnum<vi>, error out=w725:errorcluster, "FP.State"=w723:T5)
            n338 = Not Equal?(x=w723, y=w721) -> (x != y?=w722:bool)
            n339 = case shown="True" w722 {
              tunnel: [w732 w733] -> w728
              tunnel: w725 -> [w731 w733]
              tunnel: w724 -> [w730 _]
              tunnel: w721 -> [w729 _]
              frame True {
                n340 = invoke class="VI" method="FP.Open"(reference=w730, error in=w731, "State"=w729) -> (error out=w732:errorcluster)  [unwired: 2 in, 4 out]
              }
              frame False {
              }
            }
          }
        }
        n341 = call <vilib>:"Add State(s) to Queue__jki_lib_state_machine.vi"("State(s) in (\"\")"=w668) -> ("States Out"=w667:string)  [unwired: 14 in]
      }
      frame "---------- Macro ----------" {
        # "Do not put any code in this frame.\n(It is a separator no-op. You can make a copy of this frame to create a new Macro frame)"
        n342 = call <vilib>:"Add State(s) to Queue__jki_lib_state_machine.vi"("State(s) in (\"\")"=w737) -> ("States Out"=w736:string)  [unwired: 14 in]
      }
      frame "Macro: Initialize" {
        # "Initialization Macro\n(This is called once, when the VI starts)"
        n343 = call <vilib>:"Add State(s) to Queue__jki_lib_state_machine.vi"("State(s) in Front (\"\")"="UI: Cursor Set >> Busy\nData: Initialize\nInitialize Core Data\nUI: Initialize\nUI: Front Panel State >> Open\nData: Initialize Top Level\nMacro: Initialize Instruments\nMacro: Start Sweep\nUI: Cursor Set >> Idle", "State(s) in (\"\")"=w742) -> ("States Out"=w741:string)  [unwired: 13 in]
      }
      frame "Macro: Initialize Instruments" {
        # "Do not put any code in this frame.\n(It is a separator no-op. You can make a copy of this frame to create a new Macro frame)"
        n344 = call <vilib>:"Add State(s) to Queue__jki_lib_state_machine.vi"("State(s) in Front (\"\")"="Data: Initialize Instruments\nData: Disable Unsupported Instruments\nData: Open Instruments\nData: Configure Magnet Type" ("State(s) in Front (\"\")"), "State(s) in (\"\")"=w747) -> ("States Out"=w746:string)  [unwired: 13 in]
      }
      frame "Macro: Measure Instruments" {
        # "Do not put any code in this frame.\n(It is a separator no-op. You can make a copy of this frame to create a new Macro frame)"
        n345 = Unbundle By Name(w756) -> ("Instruments"=w755:T13)
        n346 = Cluster To Array(cluster=w755) -> (array=w754:refnum<class "Instrument.lvclass">[])
        n347 = for {
          tunnel: w754 -> [w765] mode=indexing
          tunnel: [w768] -> w752 mode=indexing if=w763
          tunnel: [w761] -> w750 mode=indexing
          n348 = call "Get IsConfigured.vi"("SMO"=w765) -> ("error out"=w762:errorcluster, "IsConfigured?"=w763:bool, "SMO out"=w764:refnum<class "Instrument.lvclass">)  [unwired: 8 in]
          n349 = call "Get StateName.vi"("error in (no error)"=w762, "SMO"=w764) -> ("error out"=w761:errorcluster, "StateName"=w766:string)  [unwired: 7 in, 1 out]
          n350 = Concatenate Strings("Measure: " ("string"), w766) -> (w768:string)
        }
        n351 = Merge Errors(w748, w750) -> (w749:errorcluster)
        n352 = call <vilib>:"1D String Array to Delimited String.vi"("delimiter"="\n", "string array"=w752) -> ("delimited string"=w751:string)  [unwired: 9 in]
        n353 = call <vilib>:"Add State(s) to Queue__jki_lib_state_machine.vi"("State(s) in Front (\"\")"="UI: Update Status >> reset" ("State(s) in Front (\"\")"), "State(s) at Back (\"\")"=w751) -> ("States Out"=w757:string)  [unwired: 13 in]
        n354 = call <vilib>:"Add State(s) to Queue__jki_lib_state_machine.vi"("State(s) in Front (\"\")"=w757, "State(s) in (\"\")"=w760) -> ("States Out"=w759:string)  [unwired: 13 in]
      }
      frame "Macro: Start Sweep" {
        # "Macro: Start Sweep\n()"
        n355 = call <vilib>:"Add State(s) to Queue__jki_lib_state_machine.vi"("State(s) in Front (\"\")"="Sweep: Initialize\nFile: Write JSON\nMeasure: Time\nMacro: Measure Instruments\nUI: Update AO AI Graphs >> reset\nUI: Update Lockin Graphs >> reset\nUI: Update R G Graphs\nUI: Update Lockin Graph Legend\nUI: Update Wfm Graph Legend\nUI: Update R G Graph Legend\nUI: Update Graph Axis Labels\nSweep: Start\nMeasure: DAQ\nUI: Update AO AI Graphs >> reset\nUI: Update Lockin Graphs >> reset\nUI: Update R G Graphs" ("State(s) in Front (\"\")"), "State(s) in (\"\")"=w773) -> ("States Out"=w772:string)  [unwired: 13 in]
      }
      frame "Macro: Sweep" {
        # "Template Separator\n(You can make a copy of, or modify, this frame)"
        n356 = call <vilib>:"Add State(s) to Queue__jki_lib_state_machine.vi"("State(s) in Front (\"\")"="Measure: Time\nMacro: Measure Instruments\nUI: Update AO AI Graphs\nUI: Update Lockin Graphs\nUI: Update R G Graphs\nUI: Update Timer" ("State(s) in Front (\"\")"), "State(s) in (\"\")"=w778) -> ("States Out"=w777:string)  [unwired: 13 in]
      }
      frame "Macro: Stop Sweep" {
        # "only \"return to start\"\nwhen stop button is pushed,\notherwise defer to sweep configuration"
        # "Macro: Stop Sweep\n(handle sweep finish: stop, save data, return to start)"
        n357 = Unbundle By Name(w782) -> ("UI stop"=w781:bool)
        n358 = local read "Return to Start"() -> (w779:bool)
        n359 = And(x=w781, y=w779) -> (x .and. y?=w780:bool)
        n360 = Select(t="", s=w780, f="//") -> (s? t:f=w785:string)
        n361 = Format Into String(format string="Sweep: Stop\nMeasure: DAQ Sweep\nUI: Update AO AI Graphs\nUI: Update IV Graphs\nUI: Update Graphs from wfm\nUI: Update R G Graphs\nFile: Save Lockin\n%sSweep: Return to Start" ("State(s) in Front (\"\")"), w785) -> (resulting string=w783:string)  [unwired: 2 in, 1 out]
        n362 = call <vilib>:"Add State(s) to Queue__jki_lib_state_machine.vi"("State(s) in Front (\"\")"=w783, "State(s) in (\"\")"=w790) -> ("States Out"=w789:string)  [unwired: 13 in]
      }
      frame "Macro: Exit" {
        # "Exit Macro\n(This is called once, when the VI exits)"
        n363 = Unbundle By Name(w798) -> ("Core.Close Panel on Exit?"=w797:bool)
        n364 = Select(t="UI: Front Panel State >> Close", s=w797, f="") -> (s? t:f=w794:string)
        n365 = call <vilib>:"Add State(s) to Queue__jki_lib_state_machine.vi"("State(s) in Front (\"\")"="Macro: Stop Sweep\nData: Close Instruments", "State(s) in (\"\")"=w794, "State(s) at Back (\"\")"="Data: Cleanup\nExit") -> ("States Out"=w793:string)  [unwired: 12 in]
        n366 = call <vilib>:"Add State(s) to Queue__jki_lib_state_machine.vi"("State(s) in Front (\"\")"=w793, "State(s) in (\"\")"=w801) -> ("States Out"=w800:string)  [unwired: 13 in]
      }
      frame "---------- Sweep ----------" {
        # "Do not put any code in this frame.\n(It is a separator no-op. You can make a copy of this frame to create a new Macro frame)"
        n367 = call <vilib>:"Add State(s) to Queue__jki_lib_state_machine.vi"("State(s) in (\"\")"=w805) -> ("States Out"=w804:string)  [unwired: 14 in]
      }
      frame "Sweep: Initialize" {
        # "Do not put any code in this frame.\n(It is a separator no-op. You can make a copy of this frame to create a new Macro frame)"
        n368 = Unbundle By Name(w824) -> ("Instruments.DAQ"=w821:refnum<class "Instrument.LockinAPI.lvclass">, "Transport"=w811:refnum<class "Transport.lvclass">)
        n369 = Unbundle By Name(w811) -> ("sweepTime"=w810:dbl, "initialWaitTime"=w809:dbl, "Return to Start"=w806:bool, "sweepChannels"=w808:T17, "sweepTables"=w807:cluster{"Ch":i32, "Table":dbl[]}[])
        "Sweep Time (s)" <- w810
        "Initial Wait (s)" <- w809
        "Sweep Channels" <- w808
        "Sweep Tables" <- w807
        "Return to Start" <- w806
        n370 = Bundle By Name(cluster=T10 {"sweepTime"=0.0, "initialWaitTime"=0.0, "returnToStart"=FALSE, "sweepChannels"=[]} ("Configure Sweep"), "sweepTime"=w810, "initialWaitTime"=w809, "returnToStart"=w806, "sweepChannels"=w808) -> (w822:T10)
        n371 = for {
          tunnel: [w829] -> w817 mode=indexing
          tunnel: [w828] -> w815 mode=indexing
          tunnel: w807 -> [w830] mode=indexing
          n372 = Unbundle By Name(w830) -> ("Ch"=w829:i32, "Table"=w828:dbl[])
        }
        n373 = call "Cast Lockin tsc.vi"("error in (no error)"=w818, "Instrument.LockinAPI in"=w821) -> ("error out"=w819:errorcluster, "Instrument.Lockin out"=w820:refnum<class "Instrument.Lockin.lvclass">)  [unwired: 8 in]
        n374 = call-dynamic "setSweep.vi"("error in (no error)"=w819, "Configure Sweep"=w822, "Instrument.Lockin in"=w820) -> ("error out"=w813:errorcluster, "Instrument.Lockin out"=w816:refnum<class "Instrument.Lockin.lvclass">)  [unwired: 7 in]
        n375 = call "setSweepTable.vim"("error in (no error)"=w813, "Table"=w815, "Channel"=w817, "Instrument.Lockin in"=w816) -> ("error out"=w812:errorcluster, "Instrument.Lockin out"=w814:refnum<class "Instrument.Lockin.lvclass">)  [unwired: 6 in]
        n376 = Bundle By Name(cluster=w824, "Instruments.DAQ"=w814) -> (w825:T14)
        n377 = call <vilib>:"Add State(s) to Queue__jki_lib_state_machine.vi"("State(s) in (\"\")"=w827) -> ("States Out"=w826:string)  [unwired: 14 in]
      }
      frame "Sweep: Start" {
        # "wait for sweeping to start"
        # "Do not put any code in this frame.\n(It is a separator no-op. You can make a copy of this frame to create a new Macro frame)"
        n378 = Unbundle By Name(w840) -> ("Instruments.DAQ"=w834:refnum<class "Instrument.LockinAPI.lvclass">)
        n379 = call "Cast Lockin tsc.vi"("error in (no error)"=w831, "Instrument.LockinAPI in"=w834) -> ("error out"=w832:errorcluster, "Instrument.Lockin out"=w833:refnum<class "Instrument.Lockin.lvclass">)  [unwired: 8 in]
        n380 = call-dynamic "startSweep.vi"("error in (no error)"=w832, "Instrument.Lockin in"=w833) -> ("error out"=w838:errorcluster, "Instrument.Lockin out"=w837:refnum<class "Instrument.Lockin.lvclass">)  [unwired: 8 in]
        n381 = call-dynamic "waitStatusSweepingStarted.vi"("error in (no error)"=w838, "Instrument.Lockin in"=w837) -> ("error out"=w835:errorcluster, "Instrument.Lockin out"=w836:refnum<class "Instrument.Lockin.lvclass">)  [unwired: 8 in]
        n382 = Bundle By Name(cluster=w840, "Instruments.DAQ"=w836) -> (w839:T14)
        n383 = call <vilib>:"Add State(s) to Queue__jki_lib_state_machine.vi"("State(s) in (\"\")"=w842) -> ("States Out"=w841:string)  [unwired: 14 in]
      }
      frame "Sweep: Check State" {
        # "Sweep: Check State\n(It is a separator no-op. You can make a copy of this frame to create a new Macro frame)"
        n384 = Unbundle By Name(w848) -> ("Instruments.DAQ"=w846:refnum<class "Instrument.LockinAPI.lvclass">)
        n385 = call "Cast Lockin tsc.vi"("error in (no error)"=w843, "Instrument.LockinAPI in"=w846) -> ("error out"=w844:errorcluster, "Instrument.Lockin out"=w845:refnum<class "Instrument.Lockin.lvclass">)  [unwired: 8 in]
        n386 = call-dynamic "getStatus.vi"("error in (no error)"=w844, "Instrument.Lockin"=w845) -> ("error out"=w852:errorcluster, "state"=w851:T18, "Instrument.Lockin"=w847:refnum<class "Instrument.Lockin.lvclass">)  [unwired: 7 in]
        n387 = case shown="\"sweeping\"" w851 {
          tunnel: ["Macro: Exit" ("State(s) in Front (\"\")") "Macro: Sweep" ("State(s) in Front (\"\")")] -> w850
          frame Default {
          }
          frame "sweeping" {
          }
        }
        n388 = Bundle By Name(cluster=w848, "Instruments.DAQ"=w847) -> (w849:T14)
        n389 = call <vilib>:"Add State(s) to Queue__jki_lib_state_machine.vi"("State(s) in Front (\"\")"=w850, "State(s) in (\"\")"=w854) -> ("States Out"=w853:string)  [unwired: 13 in]
      }
      frame "Sweep: Stop" {
        # "Sweep: Stop\n(It is a separator no-op. You can make a copy of this frame to create a new Macro frame)"
        n390 = Unbundle By Name(w866) -> ("Instruments.DAQ"=w860:refnum<class "Instrument.LockinAPI.lvclass">)
        n391 = call "Cast Lockin tsc.vi"("error in (no error)"=w857, "Instrument.LockinAPI in"=w860) -> ("error out"=w858:errorcluster, "Instrument.Lockin out"=w859:refnum<class "Instrument.Lockin.lvclass">)  [unwired: 8 in]
        n392 = call-dynamic "stopSweep.vi"("error in (no error)"=w858, "Instrument.Lockin in"=w859) -> ("error out"=w864:errorcluster, "Instrument.Lockin out"=w863:refnum<class "Instrument.Lockin.lvclass">)  [unwired: 8 in]
        n393 = call-dynamic "waitStatusSweepingStopped.vi"("error in (no error)"=w864, "Instrument.Lockin in"=w863) -> ("error out"=w861:errorcluster, "Instrument.Lockin out"=w862:refnum<class "Instrument.Lockin.lvclass">)  [unwired: 8 in]
        n394 = Bundle By Name(cluster=w866, "Instruments.DAQ"=w862) -> (w865:T14)
        n395 = call <vilib>:"Add State(s) to Queue__jki_lib_state_machine.vi"("State(s) in (\"\")"=w868) -> ("States Out"=w867:string)  [unwired: 14 in]
      }
      frame "Sweep: Return to Start" {
        # "Sweep: Stop\n(It is a separator no-op. You can make a copy of this frame to create a new Macro frame)"
        n396 = local read "Sweep Channels"() -> (w888:T2)
        n397 = Unbundle By Name(w890) -> ("Instruments.DAQ"=w872:refnum<class "Instrument.LockinAPI.lvclass">)
        n398 = call "Cast Lockin tsc.vi"("error in (no error)"=w869, "Instrument.LockinAPI in"=w872) -> ("error out"=w870:errorcluster, "Instrument.Lockin out"=w871:refnum<class "Instrument.Lockin.lvclass">)  [unwired: 8 in]
        n399 = call-dynamic "getAOconfig.vi"("error in (no error)"=w870, "Instrument.Lockin in"=w871) -> ("error out"=w878:errorcluster, "AOconfig"=w887:T19, "Instrument.Lockin out"=w881:refnum<class "Instrument.Lockin.lvclass">)  [unwired: 7 in]
        n400 = for {
          tunnel: w888 -> [w898] mode=indexing
          tunnel: w887 -> [w900]
          tunnel: [w895] -> w882 mode=indexing
          n401 = Unbundle By Name(w898) -> ("Channel"=w897:u16, "Start"=w896:dbl)
          n402 = Decrement(x=w897) -> (x-1=w901:u16)
          n403 = Index Array(array=w900, index=w901) -> (element=w899:T20)
          n404 = Unbundle By Name(w899) -> ("Offset"=w894:dbl)
          n405 = Bundle By Name(cluster=w898, "Start"=w894, "End"=w896, "Pattern"=Sweep.Pattern--Enum."Smooth Ramp _/") -> (w895:T3)
        }
        n406 = Bundle By Name(cluster=T10 {"sweepTime"=0.0, "initialWaitTime"=0.0, "returnToStart"=FALSE, "sweepChannels"=[]} ("Configure Sweep"), "sweepTime"=2.0 ("Sweep Time (s)"), "sweepChannels"=w882) -> (w883:T10)
        n407 = call-dynamic "setSweep.vi"("error in (no error)"=w878, "Configure Sweep"=w883, "Instrument.Lockin in"=w881) -> ("error out"=w885:errorcluster, "Instrument.Lockin out"=w886:refnum<class "Instrument.Lockin.lvclass">)  [unwired: 7 in]
        n408 = call-dynamic "startSweep.vi"("error in (no error)"=w885, "Instrument.Lockin in"=w886) -> ("error out"=w877:errorcluster, "Instrument.Lockin out"=w876:refnum<class "Instrument.Lockin.lvclass">)  [unwired: 8 in]
        n409 = call-dynamic "waitStatusSweepingStarted.vi"("error in (no error)"=w877, "Instrument.Lockin in"=w876) -> ("error out"=w874:errorcluster, "Instrument.Lockin out"=w875:refnum<class "Instrument.Lockin.lvclass">)  [unwired: 8 in]
        n410 = call-dynamic "waitStatusSweepingStopped.vi"("error in (no error)"=w874, "Instrument.Lockin in"=w875) -> ("error out"=w879:errorcluster, "Instrument.Lockin out"=w880:refnum<class "Instrument.Lockin.lvclass">)  [unwired: 8 in]
        n411 = Bundle By Name(cluster=w890, "Instruments.DAQ"=w880) -> (w889:T14)
        n412 = call <vilib>:"Add State(s) to Queue__jki_lib_state_machine.vi"("State(s) in (\"\")"=w892) -> ("States Out"=w891:string)  [unwired: 14 in]
      }
      frame "---------- Configure ----------" {
        # "Do not put any code in this frame.\n(It is a separator no-op. You can make a copy of this frame to create a new Macro frame)"
        n413 = call <vilib>:"Add State(s) to Queue__jki_lib_state_machine.vi"("State(s) in (\"\")"=w905) -> ("States Out"=w904:string)  [unwired: 14 in]
      }
      frame "Configure: Wait" {
        # "Do not put any code in this frame.\n(It is a separator no-op. You can make a copy of this frame to create a new Macro frame)"
        n414 = call <vilib>:"Add State(s) to Queue__jki_lib_state_machine.vi"("State(s) in (\"\")"=w909) -> ("States Out"=w908:string)  [unwired: 14 in]
      }
      frame "---------- Measure ----------" {
        # "Template Separator\n(You can make a copy of, or modify, this frame)"
        n415 = call <vilib>:"Add State(s) to Queue__jki_lib_state_machine.vi"("State(s) in (\"\")"=w913) -> ("States Out"=w912:string)  [unwired: 14 in]
      }
      frame "Measure: Time" {
        # "Measure: Time.\n()"
        n416 = Unbundle By Name(w917) -> ("C.E."=w919:refnum<class "Control Experiment.lvclass">)
        n417 = Get Date/Time In Seconds() -> (seconds since 1Jan1904=w922:timestamp)
        n418 = To Double Precision Float(number=w922) -> (double precision float=w914:dbl)
        n419 = call "Write Dictionary Element.vi"("error in (no error)"=w916, "value"=w914, "key"="Time", "Control Experiment in"=w919) -> ("error out"=w915:errorcluster, "Control Experiment out"=w920:refnum<class "Control Experiment.lvclass">)  [unwired: 6 in]
        n420 = Bundle By Name(cluster=w917, "C.E."=w920, "Time"=w914) -> (w921:T14)
        n421 = call <vilib>:"Add State(s) to Queue__jki_lib_state_machine.vi"("State(s) in (\"\")"=w924) -> ("States Out"=w923:string)  [unwired: 14 in]
      }
      frame "Measure: Temperature" {
        # "Measure: Temperature.\n(called dynamically if instrument is configured in Control Experiment.vi)"
        n422 = Unbundle By Name(w933) -> ("Instruments.Temperature"=w931:refnum<class "Instrument.Cryostat.lvclass">, "C.E."=w935:refnum<class "Control Experiment.lvclass">)
        n423 = call-dynamic "getTemperature.vi"("error in (no error)"=w937, "Instrument.Cryostat in"=w931) -> ("error out"=w930:errorcluster, "Temperature (K)"=w926:dbl, "Instrument.Cryostat out"=w934:refnum<class "Instrument.Cryostat.lvclass">)  [unwired: 5 in, 2 out]
        n424 = call "Write Dictionary Element.vi"("error in (no error)"=w930, "value"=w926, "key"="Temperature", "Control Experiment in"=w935) -> ("error out"=w928:errorcluster, "Control Experiment out"=w932:refnum<class "Control Experiment.lvclass">)  [unwired: 6 in]
        n425 = case shown="No Error" w928 {
          selector: w928 -> [w940 w946]
          tunnel: w926 -> [w944 _]
          tunnel: [w941 _] -> w925
          tunnel: [w940 w946] -> w927
          frame No Error {
            n426 = Format Into String(format string="T = %2f K", w944) -> (resulting string=w942:string)  [unwired: 2 in, 1 out]
            n427 = call <vilib>:"Build State String with Arguments__JKI_lib_State_Machine.vi"("Arguments (\"\")"=w942, "State"="UI: Update Status" ("format string")) -> ("State with Arguments"=w941:string)  [unwired: 4 in]
          }
          frame Error {
          }
        }
        n428 = Bundle By Name(cluster=w933, "Instruments.Temperature"=w934, "C.E."=w932, "Temperature"=w926) -> (w936:T14)
        n429 = call <vilib>:"Add State(s) to Queue__jki_lib_state_machine.vi"("State(s) in Front (\"\")"=w925, "State(s) in (\"\")"=w939) -> ("States Out"=w938:string)  [unwired: 13 in]
      }
      frame "Measure: Magnet" {
        # "Measure: Magnet.\n(called dynamically by if instrument is configured in Control Experiment.vi)"
        n430 = Unbundle By Name(w954) -> ("Instruments.Magnet"=w953:refnum<class "Instrument.Cryostat.lvclass">, "C.E."=w957:refnum<class "Control Experiment.lvclass">)
        n431 = call-dynamic "getMagnet.vi"("error in (no error)"=w956, "Instrument.Cryostat in"=w953) -> ("error out"=w952:errorcluster, "B Field (T)"=w948:dbl, "Instrument.Cryostat out"=w955:refnum<class "Instrument.Cryostat.lvclass">)  [unwired: 5 in, 2 out]
        n432 = call "Write Dictionary Element.vi"("error in (no error)"=w952, "value"=w948, "key"="Magnet", "Control Experiment in"=w957) -> ("error out"=w950:errorcluster, "Control Experiment out"=w958:refnum<class "Control Experiment.lvclass">)  [unwired: 6 in]
        n433 = case shown="No Error" w950 {
          selector: w950 -> [w962 w968]
          tunnel: w948 -> [w966 _]
          tunnel: [w963 _] -> w947
          tunnel: [w962 w968] -> w949
          frame No Error {
            n434 = Format Into String(format string="B = %2f T", w966) -> (resulting string=w964:string)  [unwired: 2 in, 1 out]
            n435 = call <vilib>:"Build State String with Arguments__JKI_lib_State_Machine.vi"("Arguments (\"\")"=w964, "State"="UI: Update Status" ("format string")) -> ("State with Arguments"=w963:string)  [unwired: 4 in]
          }
          frame Error {
          }
        }
        n436 = Bundle By Name(cluster=w954, "Instruments.Magnet"=w955, "C.E."=w958, "Magnet"=w948) -> (w959:T14)
        n437 = call <vilib>:"Add State(s) to Queue__jki_lib_state_machine.vi"("State(s) in Front (\"\")"=w947, "State(s) in (\"\")"=w961) -> ("States Out"=w960:string)  [unwired: 13 in]
      }
      frame "Measure: Vector Magnet" {
        # "Measure: Vector Magnet.\n(called dynamically by if instrument is configured in Control Experiment.vi)"
        n438 = Unbundle By Name(w980) -> ("Instruments.Magnet"=w977:refnum<class "Instrument.Cryostat.lvclass">, "C.E."=w987:refnum<class "Control Experiment.lvclass">)
        n439 = case shown="\"X\"" Magnet_Axis--Enum."Z" ("Axis") {
          tunnel: [2 ("index") 0 ("index") 1 ("index")] -> w982
          frame "Z", Default {
          }
          frame "X" {
          }
          frame "Y" {
          }
        }
        n440 = call-dynamic "getMagnetVector.vi"("error in (no error)"=w976, "Instrument.Cryostat in"=w977) -> ("error out"=w971:errorcluster, "Field (T)"=w973:dbl[], "Instrument.Cryostat out"=w975:refnum<class "Instrument.Cryostat.lvclass">)  [unwired: 5 in, 2 out]
        n441 = for {
          tunnel: w973 -> [w993] mode=indexing
          tunnel: string[] ["Bx", "By", "Bz"] ("input 1") -> [w992] mode=indexing
          shift-right: [w994] -> w986
          shift-left: w987 -> [w995]
          tunnel: w971 -> [w991]
          tunnel: [w990] -> w972
          n442 = call "Write Dictionary Element.vi"("error in (no error)"=w991, "value"=w993, "key"=w992, "Control Experiment in"=w995) -> ("error out"=w990:errorcluster, "Control Experiment out"=w994:refnum<class "Control Experiment.lvclass">)  [unwired: 6 in]
        }
        n443 = Index Array(array=w973, index #4=w982) -> (element #1=w985:dbl, element #2=w984:dbl, element #3=w983:dbl, element #4=w974:dbl)  [unwired: 3 in]
        n444 = case shown="No Error" w972 {
          selector: w972 -> [w1001 w1007]
          tunnel: w985 -> [w1005 _]
          tunnel: [w1002 _] -> w969
          tunnel: [w1001 w1007] -> w978
          tunnel: w984 -> [w1000 _]
          tunnel: w983 -> [w999 _]
          frame No Error {
            n445 = Format Into String(format string="B = [%2f, %2f, %2f]", w1005, w1000, w999) -> (resulting string=w1003:string)  [unwired: 2 in, 1 out]
            n446 = call <vilib>:"Build State String with Arguments__JKI_lib_State_Machine.vi"("Arguments (\"\")"=w1003, "State"="UI: Update Status" ("format string")) -> ("State with Arguments"=w1002:string)  [unwired: 4 in]
          }
          frame Error {
          }
        }
        n447 = Bundle By Name(cluster=w980, "Instruments.Magnet"=w975, "C.E."=w986, "Magnet"=w974) -> (w981:T14)
        n448 = call <vilib>:"Add State(s) to Queue__jki_lib_state_machine.vi"("State(s) in Front (\"\")"=w969, "State(s) in (\"\")"=w989) -> ("States Out"=w988:string)  [unwired: 13 in]
      }
      frame "Measure: Capacitance" {
        # "Measure: Capacitance.\n(called dynamically if instrument is configured in Control Experiment.vi)"
        n449 = Unbundle By Name(w1016) -> ("Instruments.Capacitance"=w1015:refnum<class "Instrument.CBridge.lvclass">, "C.E."=w1018:refnum<class "Control Experiment.lvclass">)
        n450 = call-dynamic "getCapacitance.vi"("error in (no error)"=w1017, "Instrument.CBridge in"=w1015) -> ("error out"=w1012:errorcluster, "Capacitance (pF)"=w1011:dbl, "Instrument.CBridge out"=w1014:refnum<class "Instrument.CBridge.lvclass">)  [unwired: 7 in]
        n451 = call "Write Dictionary Element.vi"("error in (no error)"=w1012, "value"=w1011, "key"="Capacitance", "Control Experiment in"=w1018) -> ("error out"=w1010:errorcluster, "Control Experiment out"=w1019:refnum<class "Control Experiment.lvclass">)  [unwired: 6 in]
        n452 = case shown="No Error" w1010 {
          selector: w1010 -> [w1023 w1029]
          tunnel: w1011 -> [w1027 _]
          tunnel: [w1024 _] -> w1008
          tunnel: [w1023 w1029] -> w1009
          frame No Error {
            n453 = Format Into String(format string="C = %2f pF", w1027) -> (resulting string=w1025:string)  [unwired: 2 in, 1 out]
            n454 = call <vilib>:"Build State String with Arguments__JKI_lib_State_Machine.vi"("Arguments (\"\")"=w1025, "State"="UI: Update Status" ("format string")) -> ("State with Arguments"=w1024:string)  [unwired: 4 in]
          }
          frame Error {
          }
        }
        n455 = Bundle By Name(cluster=w1016, "Instruments.Capacitance"=w1014, "C.E."=w1019) -> (w1020:T14)
        n456 = call <vilib>:"Add State(s) to Queue__jki_lib_state_machine.vi"("State(s) in Front (\"\")"=w1008, "State(s) in (\"\")"=w1022) -> ("States Out"=w1021:string)  [unwired: 13 in]
      }
      frame "Measure: Strain Cell" {
        # "Measure: Strain Cell.\n(called dynamically if instrument is configured in Control Experiment.vi)"
        n457 = Unbundle By Name(w1038) -> ("Instruments.Strain Cell"=w1037:refnum<class "Instrument.Strain.lvclass">, "C.E."=w1040:refnum<class "Control Experiment.lvclass">)
        n458 = call-dynamic "getStrain.vi"("error in (no error)"=w1039, "Instrument.Strain in"=w1037) -> ("error out"=w1034:errorcluster, "Strain (V)"=w1030:dbl, "Instrument.Strain out"=w1036:refnum<class "Instrument.Strain.lvclass">)  [unwired: 7 in]
        n459 = call "Write Dictionary Element.vi"("error in (no error)"=w1034, "value"=w1030, "key"="Strain", "Control Experiment in"=w1040) -> ("error out"=w1033:errorcluster, "Control Experiment out"=w1041:refnum<class "Control Experiment.lvclass">)  [unwired: 6 in]
        n460 = case shown="No Error" w1033 {
          selector: w1033 -> [w1045 w1051]
          tunnel: w1030 -> [w1049 _]
          tunnel: [w1046 _] -> w1031
          tunnel: [w1045 w1051] -> w1032
          frame No Error {
            n461 = Format Into String(format string="Strain = %2f V", w1049) -> (resulting string=w1047:string)  [unwired: 2 in, 1 out]
            n462 = call <vilib>:"Build State String with Arguments__JKI_lib_State_Machine.vi"("Arguments (\"\")"=w1047, "State"="UI: Update Status" ("format string")) -> ("State with Arguments"=w1046:string)  [unwired: 4 in]
          }
          frame Error {
          }
        }
        n463 = Bundle By Name(cluster=w1038, "Instruments.Strain Cell"=w1036, "C.E."=w1041) -> (w1042:T14)
        n464 = call <vilib>:"Add State(s) to Queue__jki_lib_state_machine.vi"("State(s) in Front (\"\")"=w1031, "State(s) in (\"\")"=w1044) -> ("States Out"=w1043:string)  [unwired: 13 in]
      }
      frame "Measure: Delay Line" {
        # "Measure: Delay Line.\n(called dynamically if instrument is configured in Control Experiment.vi)"
        n465 = Unbundle By Name(w1060) -> ("Instruments.Delay Line"=w1059:refnum<class "Instrument.DelayLine.lvclass">, "C.E."=w1062:refnum<class "Control Experiment.lvclass">)
        n466 = call-dynamic "getDelay.vi"("error in (no error)"=w1061, "Instrument.DelayLine in"=w1059) -> ("error out"=w1056:errorcluster, "delay (ps)"=w1052:dbl, "Instrument.DelayLine out"=w1058:refnum<class "Instrument.DelayLine.lvclass">)  [unwired: 6 in, 1 out]
        n467 = call "Write Dictionary Element.vi"("error in (no error)"=w1056, "value"=w1052, "key"="Delay", "Control Experiment in"=w1062) -> ("error out"=w1055:errorcluster, "Control Experiment out"=w1063:refnum<class "Control Experiment.lvclass">)  [unwired: 6 in]
        n468 = case shown="No Error" w1055 {
          selector: w1055 -> [w1067 w1073]
          tunnel: w1052 -> [w1071 _]
          tunnel: [w1068 _] -> w1053
          tunnel: [w1067 w1073] -> w1054
          frame No Error {
            n469 = Format Into String(format string="Delay = %2f ps", w1071) -> (resulting string=w1069:string)  [unwired: 2 in, 1 out]
            n470 = call <vilib>:"Build State String with Arguments__JKI_lib_State_Machine.vi"("Arguments (\"\")"=w1069, "State"="UI: Update Status" ("format string")) -> ("State with Arguments"=w1068:string)  [unwired: 4 in]
          }
          frame Error {
          }
        }
        n471 = Bundle By Name(cluster=w1060, "Instruments.Delay Line"=w1058, "C.E."=w1063) -> (w1064:T14)
        n472 = call <vilib>:"Add State(s) to Queue__jki_lib_state_machine.vi"("State(s) in Front (\"\")"=w1053, "State(s) in (\"\")"=w1066) -> ("States Out"=w1065:string)  [unwired: 13 in]
      }
      frame "Measure: Rotator" {
        # "Measure: Delay Line.\n(called dynamically if instrument is configured in Control Experiment.vi)"
        n473 = Unbundle By Name(w1082) -> ("Instruments.Rotator"=w1081:refnum<class "Instrument.Cryostat.lvclass">, "C.E."=w1084:refnum<class "Control Experiment.lvclass">)
        n474 = call-dynamic "getAngle.vi"("error in (no error)"=w1083, "Instrument.Cryostat in"=w1081) -> ("error out"=w1078:errorcluster, "Angle (°)"=w1074:dbl, "Instrument.Cryostat out"=w1080:refnum<class "Instrument.Cryostat.lvclass">)  [unwired: 5 in, 2 out]
        n475 = call "Write Dictionary Element.vi"("error in (no error)"=w1078, "value"=w1074, "key"="Angle", "Control Experiment in"=w1084) -> ("error out"=w1077:errorcluster, "Control Experiment out"=w1085:refnum<class "Control Experiment.lvclass">)  [unwired: 6 in]
        n476 = case shown="No Error" w1077 {
          selector: w1077 -> [w1089 w1095]
          tunnel: w1074 -> [w1093 _]
          tunnel: [w1090 _] -> w1075
          tunnel: [w1089 w1095] -> w1076
          frame No Error {
            n477 = Format Into String(format string="Angle = %2f°", w1093) -> (resulting string=w1091:string)  [unwired: 2 in, 1 out]
            n478 = call <vilib>:"Build State String with Arguments__JKI_lib_State_Machine.vi"("Arguments (\"\")"=w1091, "State"="UI: Update Status" ("format string")) -> ("State with Arguments"=w1090:string)  [unwired: 4 in]
          }
          frame Error {
          }
        }
        n479 = Bundle By Name(cluster=w1082, "Instruments.Rotator"=w1080, "C.E."=w1085) -> (w1086:T14)
        n480 = call <vilib>:"Add State(s) to Queue__jki_lib_state_machine.vi"("State(s) in Front (\"\")"=w1075, "State(s) in (\"\")"=w1088) -> ("States Out"=w1087:string)  [unwired: 13 in]
      }
      frame "Measure: DAQ" {
        # "Gives the AI and AO waveform which refreshes as per the Lockin sampling parameters"
        # "Measure Lockin\n(Read intermediate values of the waveforms)"
        n481 = Unbundle By Name(w1112) -> ("Instruments.DAQ"=w1099:refnum<class "Instrument.LockinAPI.lvclass">)
        n482 = local read "Sweep Channels"() -> (w1102:T2)
        n483 = call "Cast Lockin tsc.vi"("error in (no error)"=w1096, "Instrument.LockinAPI in"=w1099) -> ("error out"=w1097:errorcluster, "Instrument.Lockin out"=w1098:refnum<class "Instrument.Lockin.lvclass">)  [unwired: 8 in]
        n484 = for {
          tunnel: [w1121] -> w1101
          tunnel: w1102 -> [w1124] mode=indexing
          stop <- w1123 stop-if-true
          # "find the 1st enabled channel"
          n485 = Unbundle By Name(w1124) -> ("Enable?"=w1123:bool, "Channel"=w1122:u16)
          n486 = Decrement(x=w1122) -> (x-1=w1121:u16)
        }
        n487 = call-dynamic "getAOconfig.vi"("error in (no error)"=w1097, "Instrument.Lockin in"=w1098) -> ("error out"=w1104:errorcluster, "AOconfig"=w1100:T19, "Instrument.Lockin out"=w1107:refnum<class "Instrument.Lockin.lvclass">)  [unwired: 7 in]
        n488 = call-dynamic "getAOwfm.vi"("error in (no error)"=w1104, "Instrument.Lockin in"=w1107) -> ("error out"=w1114:errorcluster, "AO Waveforrm"=w1108:waveform(dbl)[], "Instrument.Lockin out"=w1116:refnum<class "Instrument.Lockin.lvclass">)  [unwired: 7 in]
        n489 = call-dynamic "getAIwfm.vi"("error in (no error)"=w1114, "Instrument.Lockin in"=w1116) -> ("error out"=w1113:errorcluster, "AI Waveform"=w1109:waveform(dbl)[], "Instrument.Lockin out"=w1115:refnum<class "Instrument.Lockin.lvclass">)  [unwired: 7 in]
        n490 = Index Array(array=w1100, index=w1101) -> (element=w1106:T20)
        n491 = for {
          tunnel: [w1126] -> w1103 mode=indexing
          tunnel: w1100 -> [w1125] mode=indexing
          n492 = Unbundle By Name(w1125) -> ("Amplitude"=w1126:dbl)
        }
        n493 = call-dynamic "getResults.vi"("error in (no error)"=w1113, "Instrument.Lockin in"=w1115) -> ("error out"=w1118:errorcluster, "Results (Dictionary)"=w1117:cluster{"key":string, "value":dbl}[], "Instrument.Lockin out"=w1110:refnum<class "Instrument.Lockin.lvclass">)  [unwired: 6 in, 1 out]
        n494 = Unbundle By Name(w1106) -> ("Offset"=w1105:dbl)
        n495 = Bundle By Name(cluster=w1112, "Instruments.DAQ"=w1110, "Results (Dictionary)"=w1117, "AI Waveform"=w1109, "AO Waveforrm"=w1108, "Amplitude"=w1103, "Sweep Value"=w1105) -> (w1111:T14)
        n496 = call <vilib>:"Add State(s) to Queue__jki_lib_state_machine.vi"("State(s) in (\"\")"=w1120) -> ("States Out"=w1119:string)  [unwired: 14 in]
      }
      frame "Measure: DAQ Sweep" {
        # "Gives the AI and AO waveform which refreshes as per the Lockin sampling parameters"
        # "Measure: Lockin Sweep\n(get all sweep waveforms from lockin)"
        n497 = Unbundle By Name(w1139) -> ("Instruments.DAQ"=w1130:refnum<class "Instrument.LockinAPI.lvclass">)
        n498 = call "Cast Lockin tsc.vi"("error in (no error)"=w1127, "Instrument.LockinAPI in"=w1130) -> ("error out"=w1128:errorcluster, "Instrument.Lockin out"=w1129:refnum<class "Instrument.Lockin.lvclass">)  [unwired: 8 in]
        n499 = call-dynamic "getSweepData.vi"("error in (no error)"=w1128, "Instrument.Lockin in"=w1129) -> ("error out"=w1136:errorcluster, "SweepData"=w1131:T22, "Instrument.Lockin out"=w1137:refnum<class "Instrument.Lockin.lvclass">)  [unwired: 7 in]
        n500 = Unbundle By Name(w1131) -> ("AO"=w1135:waveform(dbl)[], "AI"=w1134:waveform(dbl)[], "X"=w1133:waveform(dbl)[], "Y"=w1132:waveform(dbl)[])
        n501 = Bundle By Name(cluster=w1139, "Instruments.DAQ"=w1137, "Sweep_AO"=w1135, "Sweep_AI"=w1134, "Sweep_X"=w1133, "Sweep_Y"=w1132) -> (w1138:T14)
        n502 = call <vilib>:"Add State(s) to Queue__jki_lib_state_machine.vi"("State(s) in (\"\")"=w1141) -> ("States Out"=w1140:string)  [unwired: 14 in]
      }
      frame "---------- File ----------" {
        # "Template Separator\n(You can make a copy of, or modify, this frame)"
        n503 = call <vilib>:"Add State(s) to Queue__jki_lib_state_machine.vi"("State(s) in (\"\")"=w1145) -> ("States Out"=w1144:string)  [unwired: 14 in]
      }
      frame "File: Configure" {
        # "Template Separator\n(You can make a copy of, or modify, this frame)"
        n504 = call <vilib>:"Add State(s) to Queue__jki_lib_state_machine.vi"("State(s) in (\"\")"=w1149) -> ("States Out"=w1148:string)  [unwired: 14 in]
      }
      frame "File: Write JSON" {
        # "Template Separator\n(You can make a copy of, or modify, this frame)"
        n505 = Unbundle By Name(w1157) -> ("C.E."=w1155:refnum<class "Control Experiment.lvclass">)
        n506 = call "Write JSON to Dictionary.vi"("error in (no error)"=w1152, "Control Experiment in"=w1155) -> ("error out"=w1153:errorcluster, "Control Experiment out"=w1154:refnum<class "Control Experiment.lvclass">)  [unwired: 8 in]
        n507 = local read "Sweep Time (s)"() -> (w1164:dbl)
        n508 = local read "Initial Wait (s)"() -> (w1165:dbl)
        n509 = local read "Return to Start"() -> (w1166:bool)
        n510 = local read "Sweep Channels"() -> (w1167:T2)
        n511 = local read "Sweep Tables"() -> (w1150:cluster{"Ch":i32, "Table":dbl[]}[])
        n512 = Bundle By Name(cluster=T12 {"initialWaitTime"=0.0, "sweepTime"=0.0, "Return to Start"=FALSE, "sweepChannels"=[], "sweepTables"=[]} ("Lockin_Sweep"), "sweepTime"=w1164, "initialWaitTime"=w1165, "Return to Start"=w1166, "sweepChannels"=w1167, "sweepTables"=w1150) -> (w1162:T12)
        n513 = call "To JSON Text.vim"("error in (no error)"=w1153, "Anything"=w1162) -> ("error out"=w1156:errorcluster, "<JSON>"=w1163:string)  [unwired: 8 in]
        n514 = call "Write Dictionary Element.vi"("error in (no error)"=w1156, "value"=w1163, "key"="<LockinSweep>", "Control Experiment in"=w1154) -> ("error out"=w1160:errorcluster, "Control Experiment out"=w1159:refnum<class "Control Experiment.lvclass">)  [unwired: 6 in]
        n515 = Bundle By Name(cluster=w1157, "C.E."=w1159) -> (w1158:T14)
        n516 = call <vilib>:"Add State(s) to Queue__jki_lib_state_machine.vi"("State(s) in (\"\")"=w1169) -> ("States Out"=w1168:string)  [unwired: 14 in]
      }
      frame "File: Save Lockin" {
        # "F --> create\nnew file\neach time\nthis state runs"
        # "build cluster array(s) of multiple 1D data, dynamically name waves"
        # "Template Separator\n(You can make a copy of, or modify, this frame)"
        n517 = Unbundle By Name(w1183) -> ("C.E."=w1186:refnum<class "Control Experiment.lvclass">, "Sweep_AO"=w1175:waveform(dbl)[], "Sweep_AI"=w1174:waveform(dbl)[], "Sweep_X"=w1173:waveform(dbl)[], "Sweep_Y"=w1177:waveform(dbl)[])
        n518 = Build Cluster Array(w1175, w1174, w1173, w1177) -> (w1170:cluster{"Sweep_Y":waveform(dbl)[]}[])
        n519 = for {
          shift-right: [w1193] -> w1178
          shift-left: w1176 -> [w1194]
          tunnel: string[] ["AO", "AI", "X", "Y"] -> [w1192] mode=indexing
          tunnel: [w1191] -> w1171 mode=concatenating
          tunnel: w1170 -> [w1190] mode=indexing
          n520 = Unbundle(w1190) -> ("Sweep_Y"=w1189:waveform(dbl)[])
          n521 = call "Data to Dictionary.vim"("Error in"=w1194, "Data in"=w1189, "Label in"=w1192) -> ("Error out"=w1193:errorcluster, "Data out"=w1191:T23[])  [unwired: 7 in]
        }
        n522 = call "Write Dictionary Elements (Loop).vi"("error in (no error)"=w1178, "Data in"=w1171, "Control Experiment in"=w1186) -> ("error out"=w1180:errorcluster, "Control Experiment out"=w1182:refnum<class "Control Experiment.lvclass">)  [unwired: 7 in]
        n523 = call "Save Transport TDMS File.vi"("append?"=FALSE, "error in (no error)"=w1180, "Control Experiment in"=w1182) -> ("error out"=w1181:errorcluster, "Control Experiment out"=w1185:refnum<class "Control Experiment.lvclass">)  [unwired: 7 in]
        n524 = Bundle By Name(cluster=w1183, "C.E."=w1185) -> (w1184:T14)
        n525 = call <vilib>:"Add State(s) to Queue__jki_lib_state_machine.vi"("State(s) in (\"\")"=w1188) -> ("States Out"=w1187:string)  [unwired: 14 in]
      }
    }
  }
  "error out" <- w2
  n526 = Unbundle By Name(w4) -> ("Transport"=→"Transport out":refnum<class "Transport.lvclass">)
